vi "Time.vi"(8 "error in (no error)":errorcluster, 10 "Control In":T2={"I-O.lvclass"=refnum, "Gantry"=refnum, "Dispenser"="COM1"}, 11 "Sensor Dispense in":refnum<class "Sensor Dispense.lvclass">) -> (0 "error out":errorcluster, 1 "Timing Data":i32[](array[numeric]), 2 "Control Out":T2={"I-O.lvclass"=refnum, "Gantry"=refnum, "Dispenser"="COM1"}, 3 "Sensor Dispense out":refnum<class "Sensor Dispense.lvclass">)   [LabVIEW 2021, in "Sensor Dispense.lvclass"]
uses:
  Projects/Sensor Dispense.lvclass
  C:/Users/HEP/Documents/GitHub/Gantry/UCSB-Gantry-HEP-main/Classes/Routine/Dispense/Dispense.lvclass
  Controller/Controllers.ctl
  Controller/I-O/I-O.lvclass
  C:/Program Files (x86)/Aerotech/A3200/LabVIEW/2010/Bin/Aerotech.A3200.dll
  Program Files (x86)/Aerotech/A3200/LabVIEW/2010/Bin/Aerotech.A3200.dll
  TypeOfHexaboard.ctl
  Projects/Sensor Dispense.lvclass/Sensor Dispense.ctl
  Controller/Motion/Motion.lvclass
  Controller/Motion/A3200/A3200.lvclass
  Controller/Controller.lvclass
  Routine.lvclass
panel:
  in  "Type of Hexaboard":T1
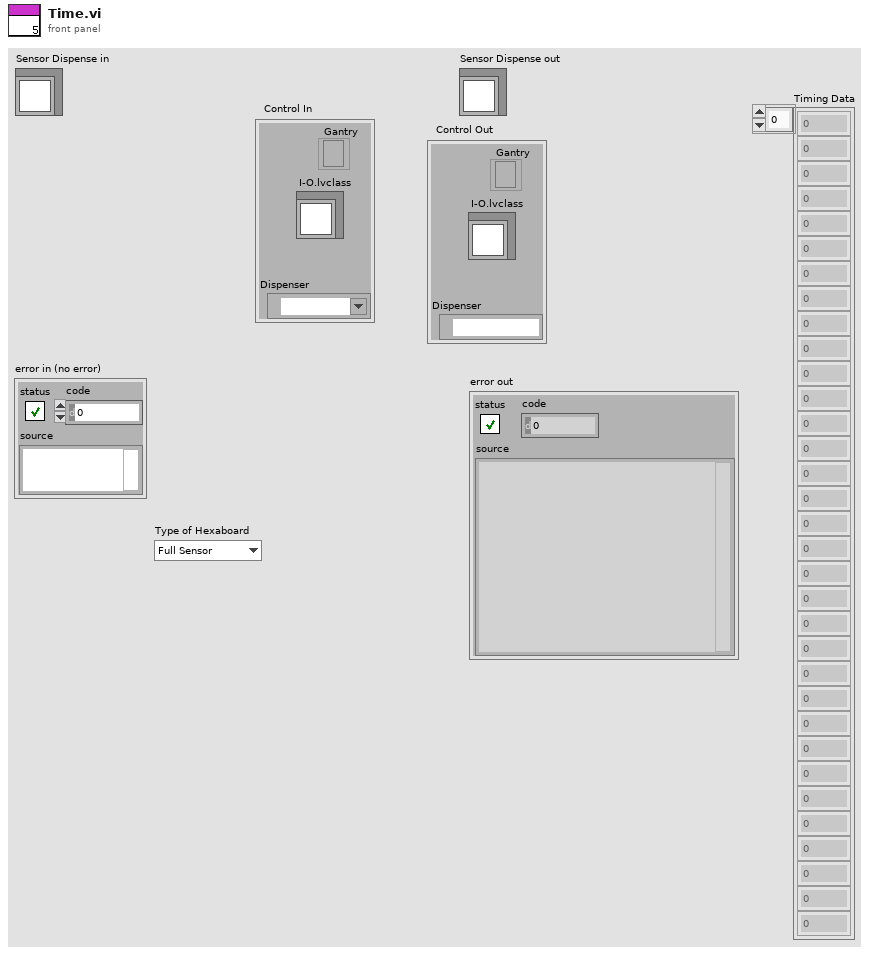
[diagram p1: front panel]
types:
  T1 = typedef "Routine.lvclass/TypeOfHexaboard.ctl" = enum16{"Full Sensor", "Full PCB", "Right Partial PCB", "Right Partial Sensor", "Al Dummy Right Partial Sensor"}
  T2 = typedef "Controller.lvclass/Controllers.ctl" = cluster{"I-O.lvclass":refnum<class "I-O.lvclass">, "Gantry":refnum<k24>, "Dispenser":refnum<visa-resource-name>}
  T3 = cluster{"Endpoints":dbl[][], "Center":dbl[], "CW/CCW":dbl, "Dispense Type":enum16{"N-gon", "Square", "Arc", "Dot", "Line", "Circle"}}[]
  T4 = cluster{"Endpoints":dbl[][], "Center":dbl[], "CW/CCW":dbl, "Dispense Type":enum16{"N-gon", "Square", "Arc", "Dot", "Line", "Circle"}}
  T5 = enum16{"N-gon", "Square", "Arc", "Dot", "Line", "Circle"}
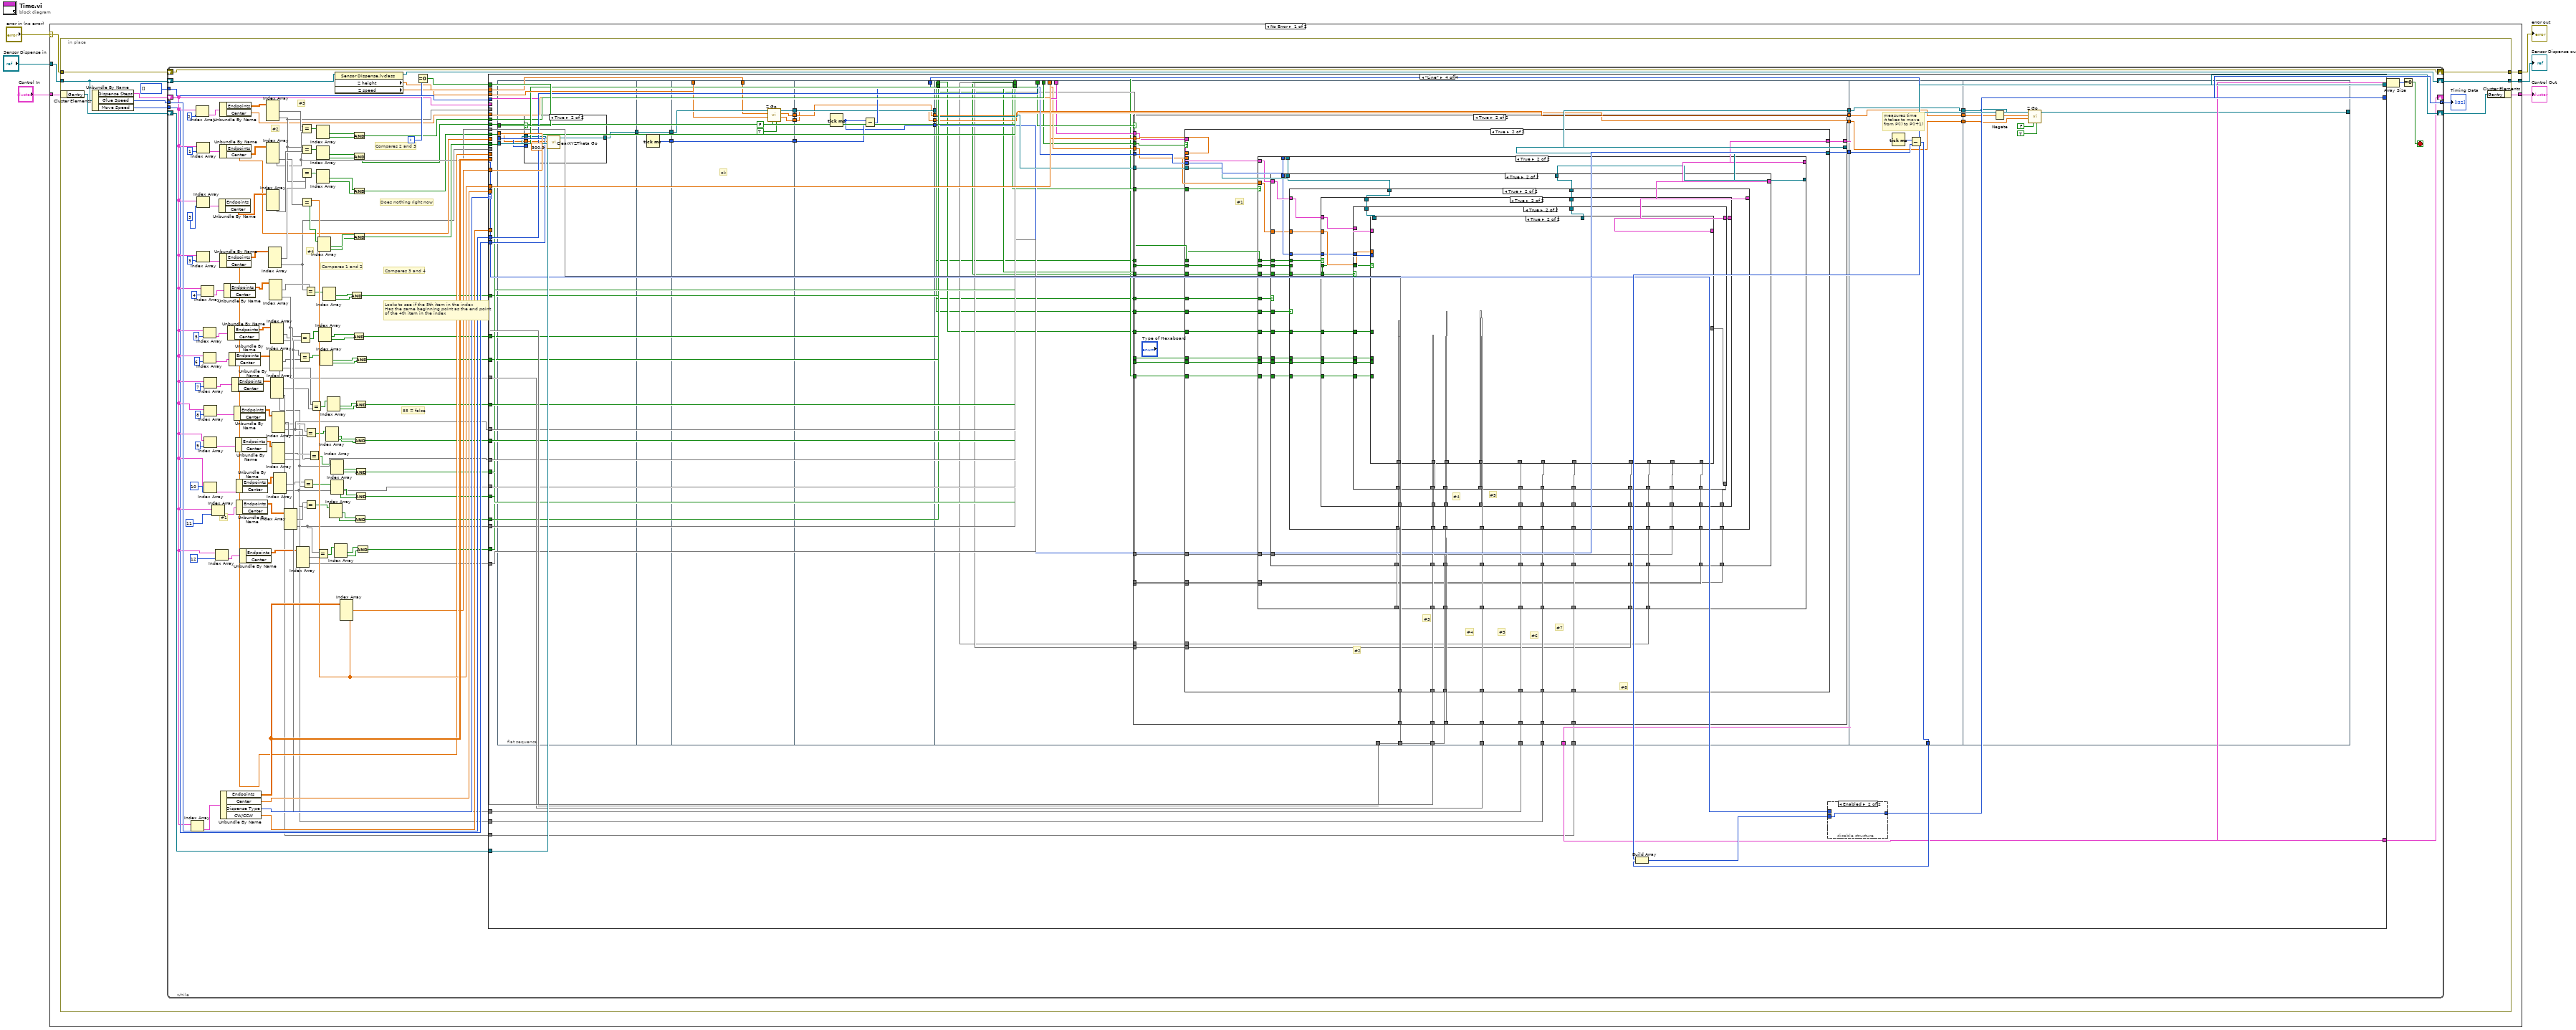
[diagram p0: block diagram]
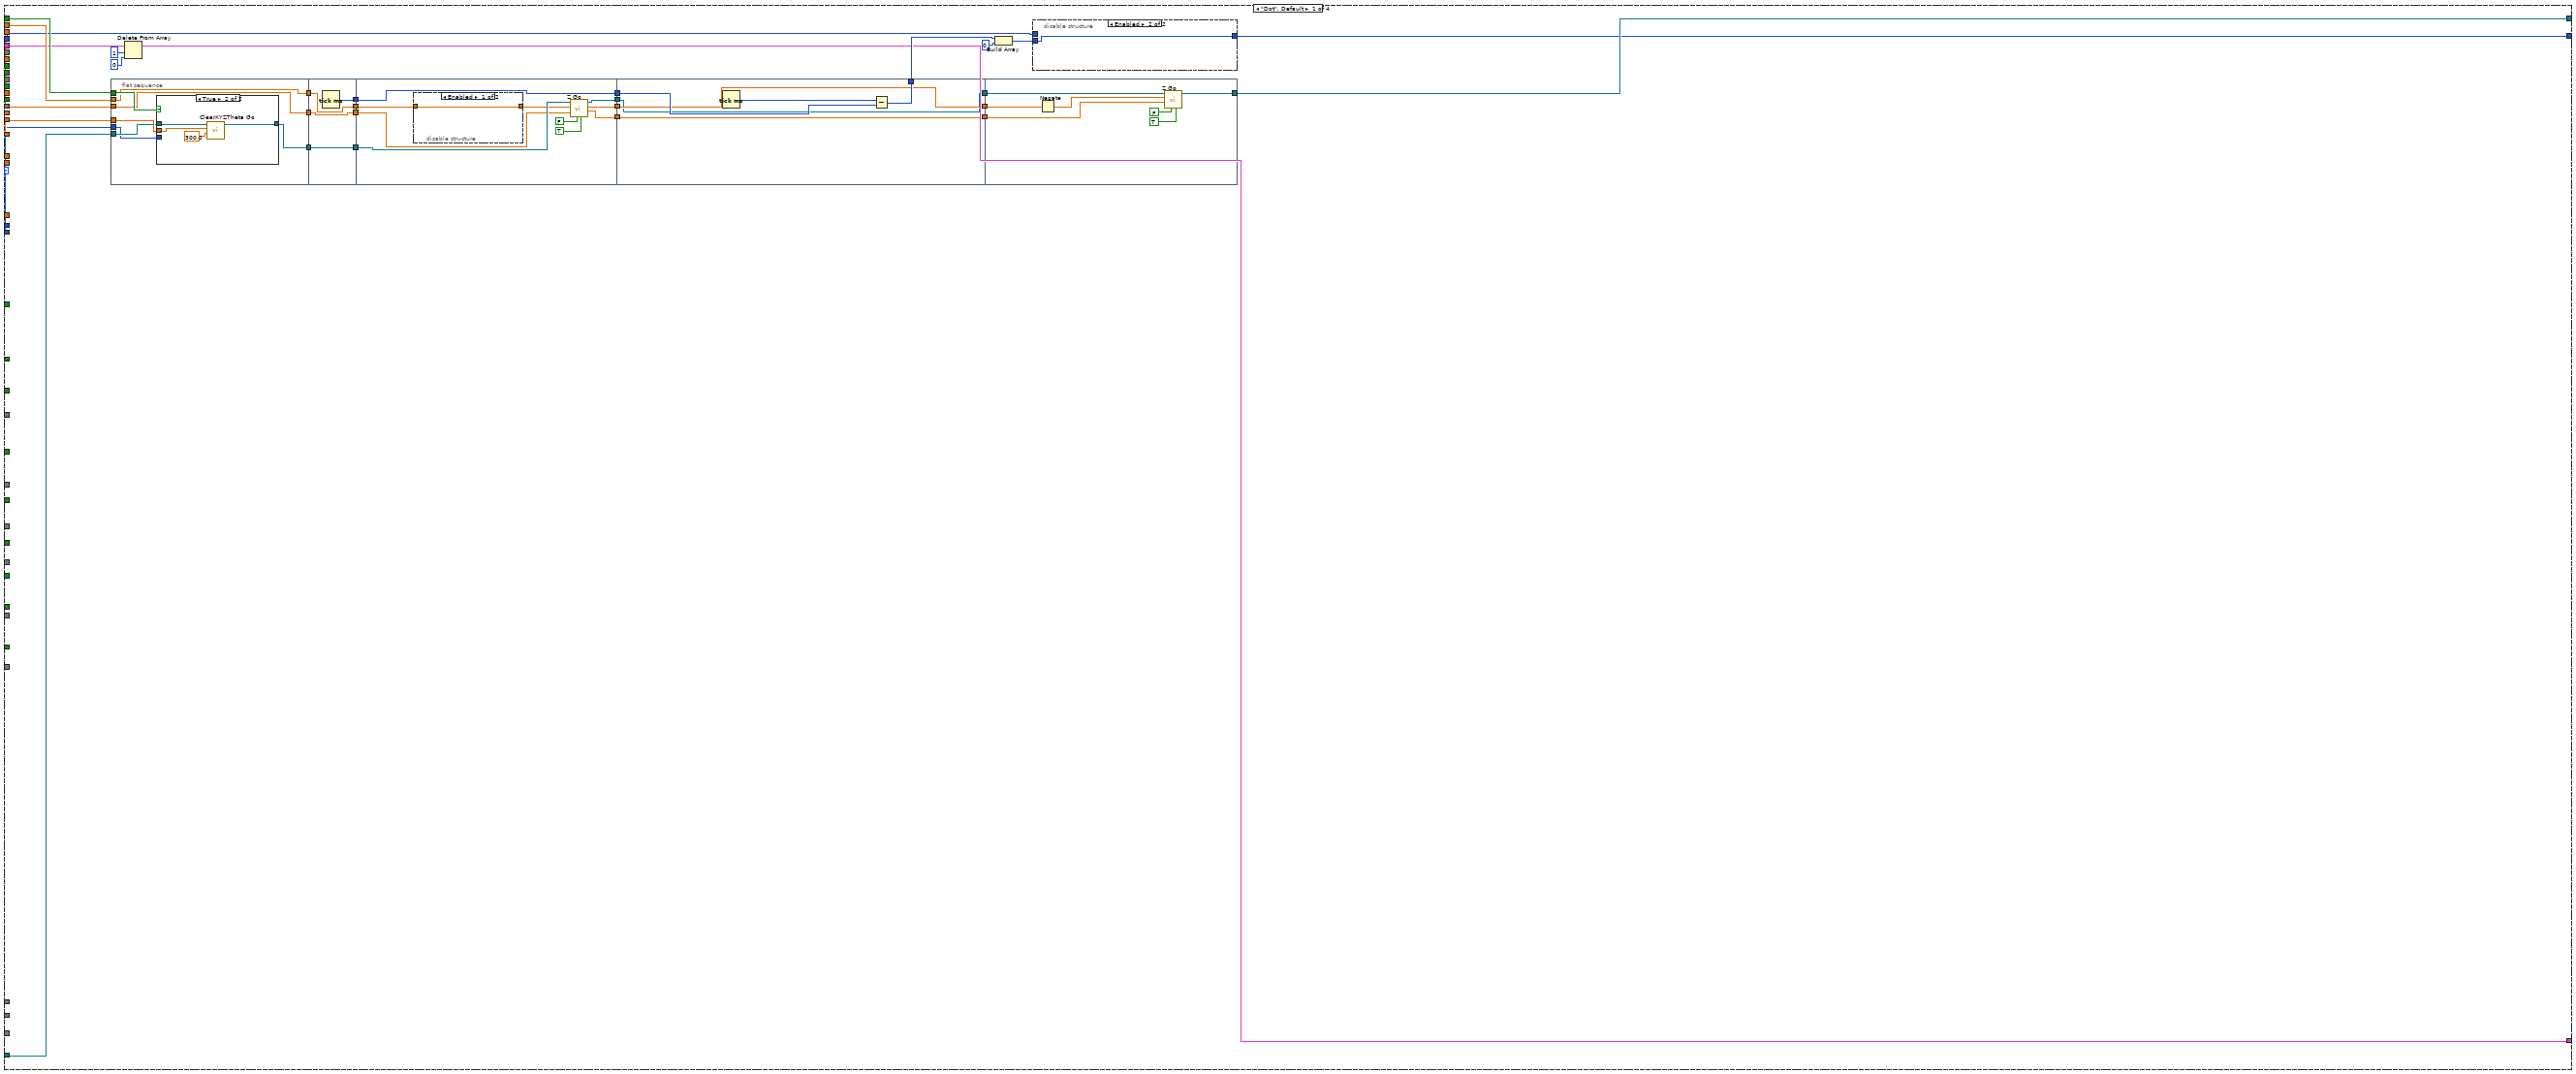
[diagram p2: hidden frame]
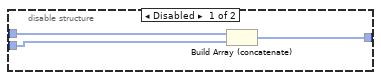
[diagram p3: hidden frame]
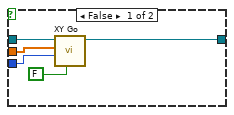
[diagram p4: hidden frame]
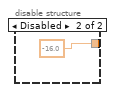
[diagram p5: hidden frame]
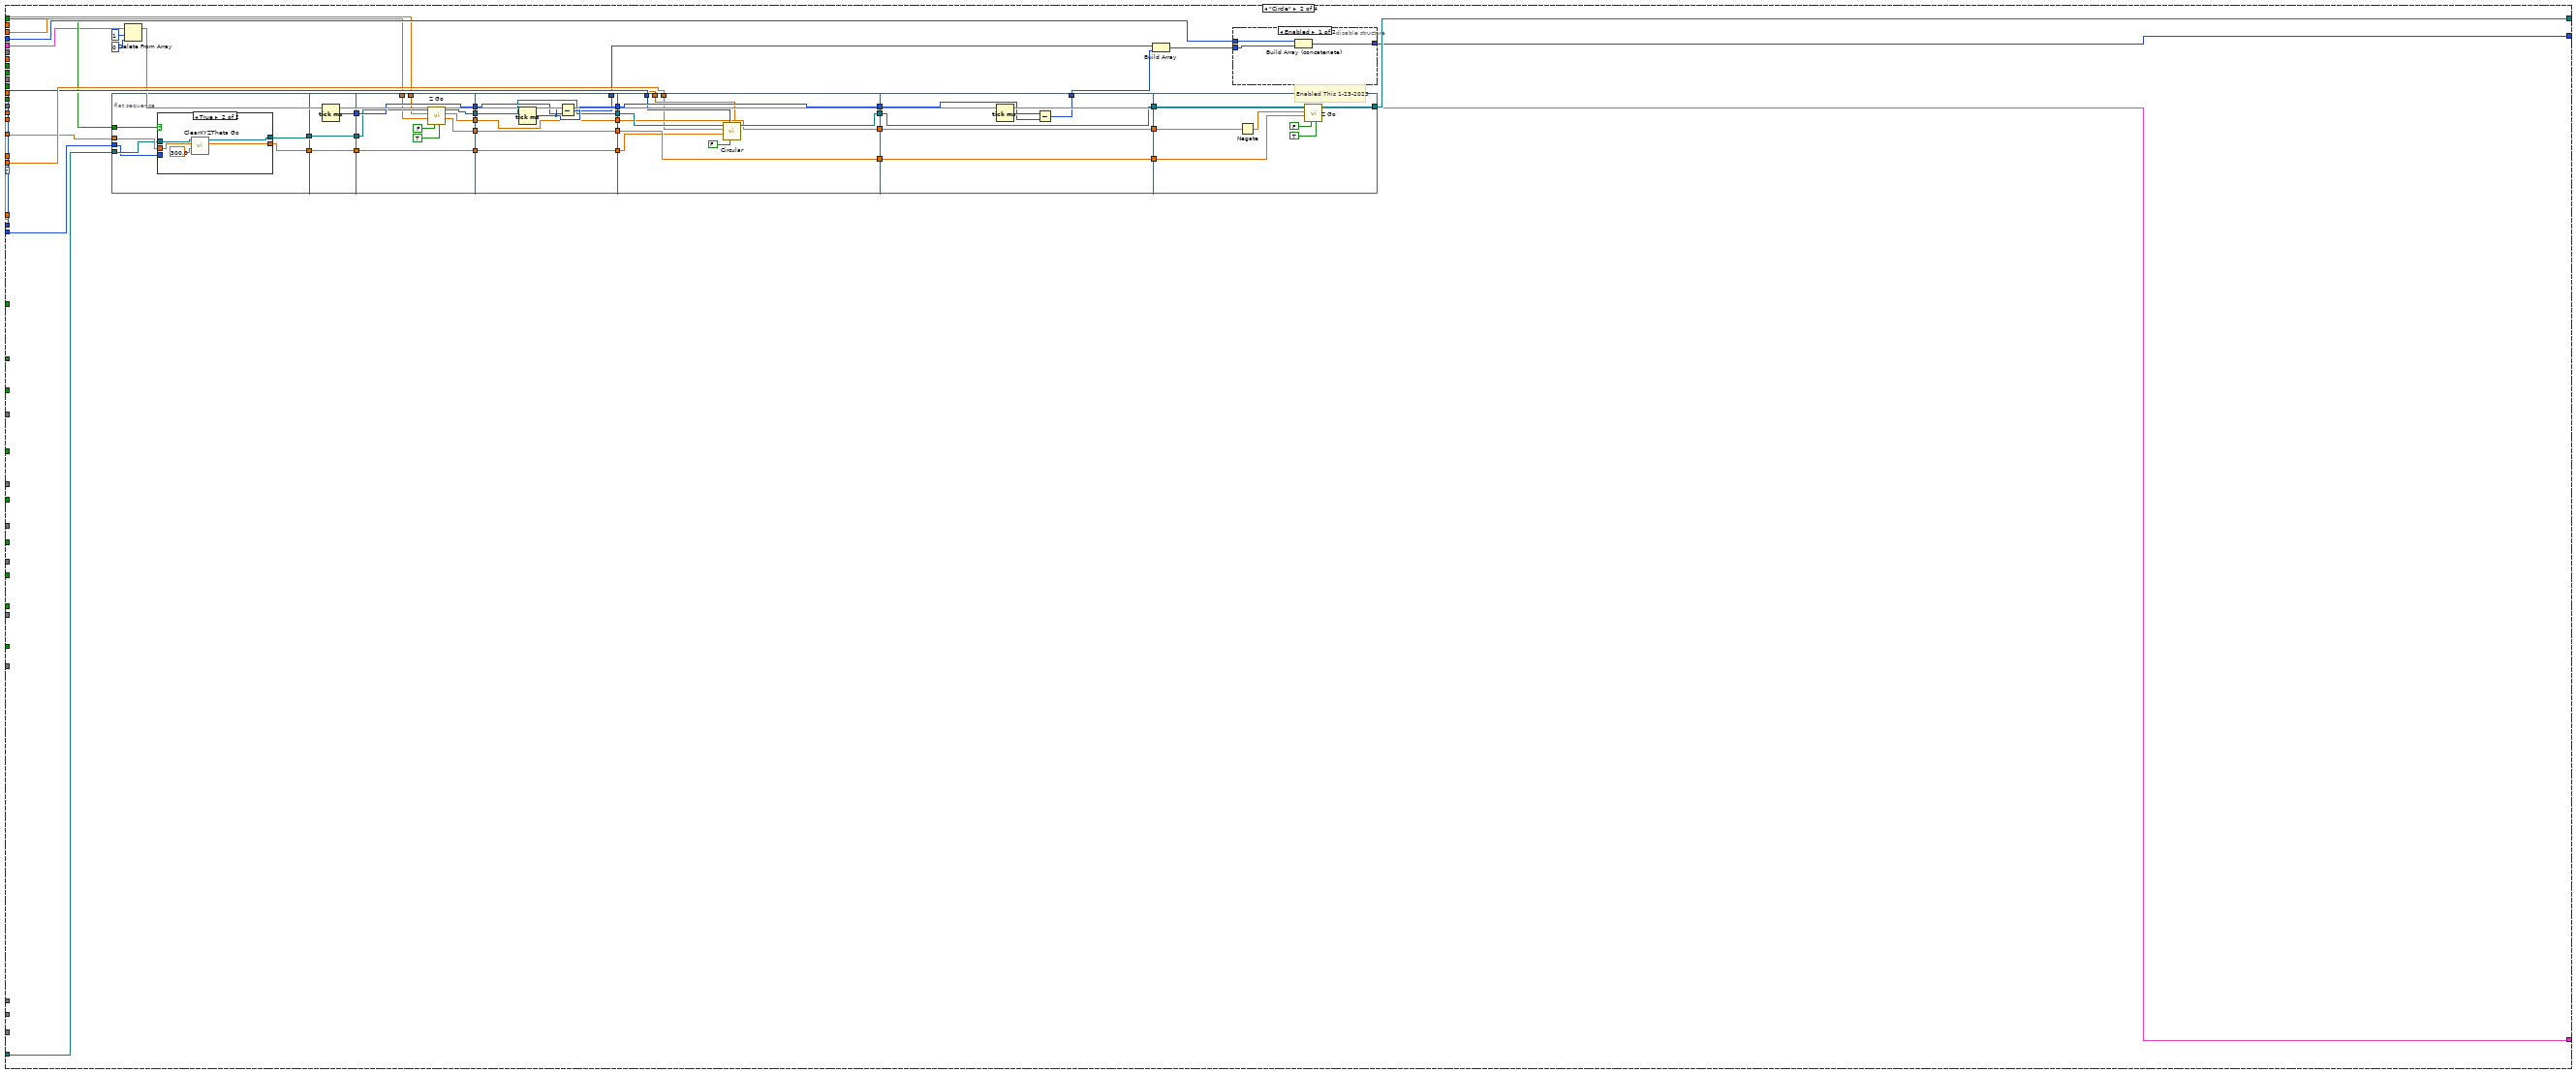
[diagram p6: hidden frame]
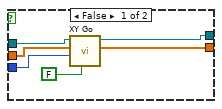
[diagram p8: hidden frame]
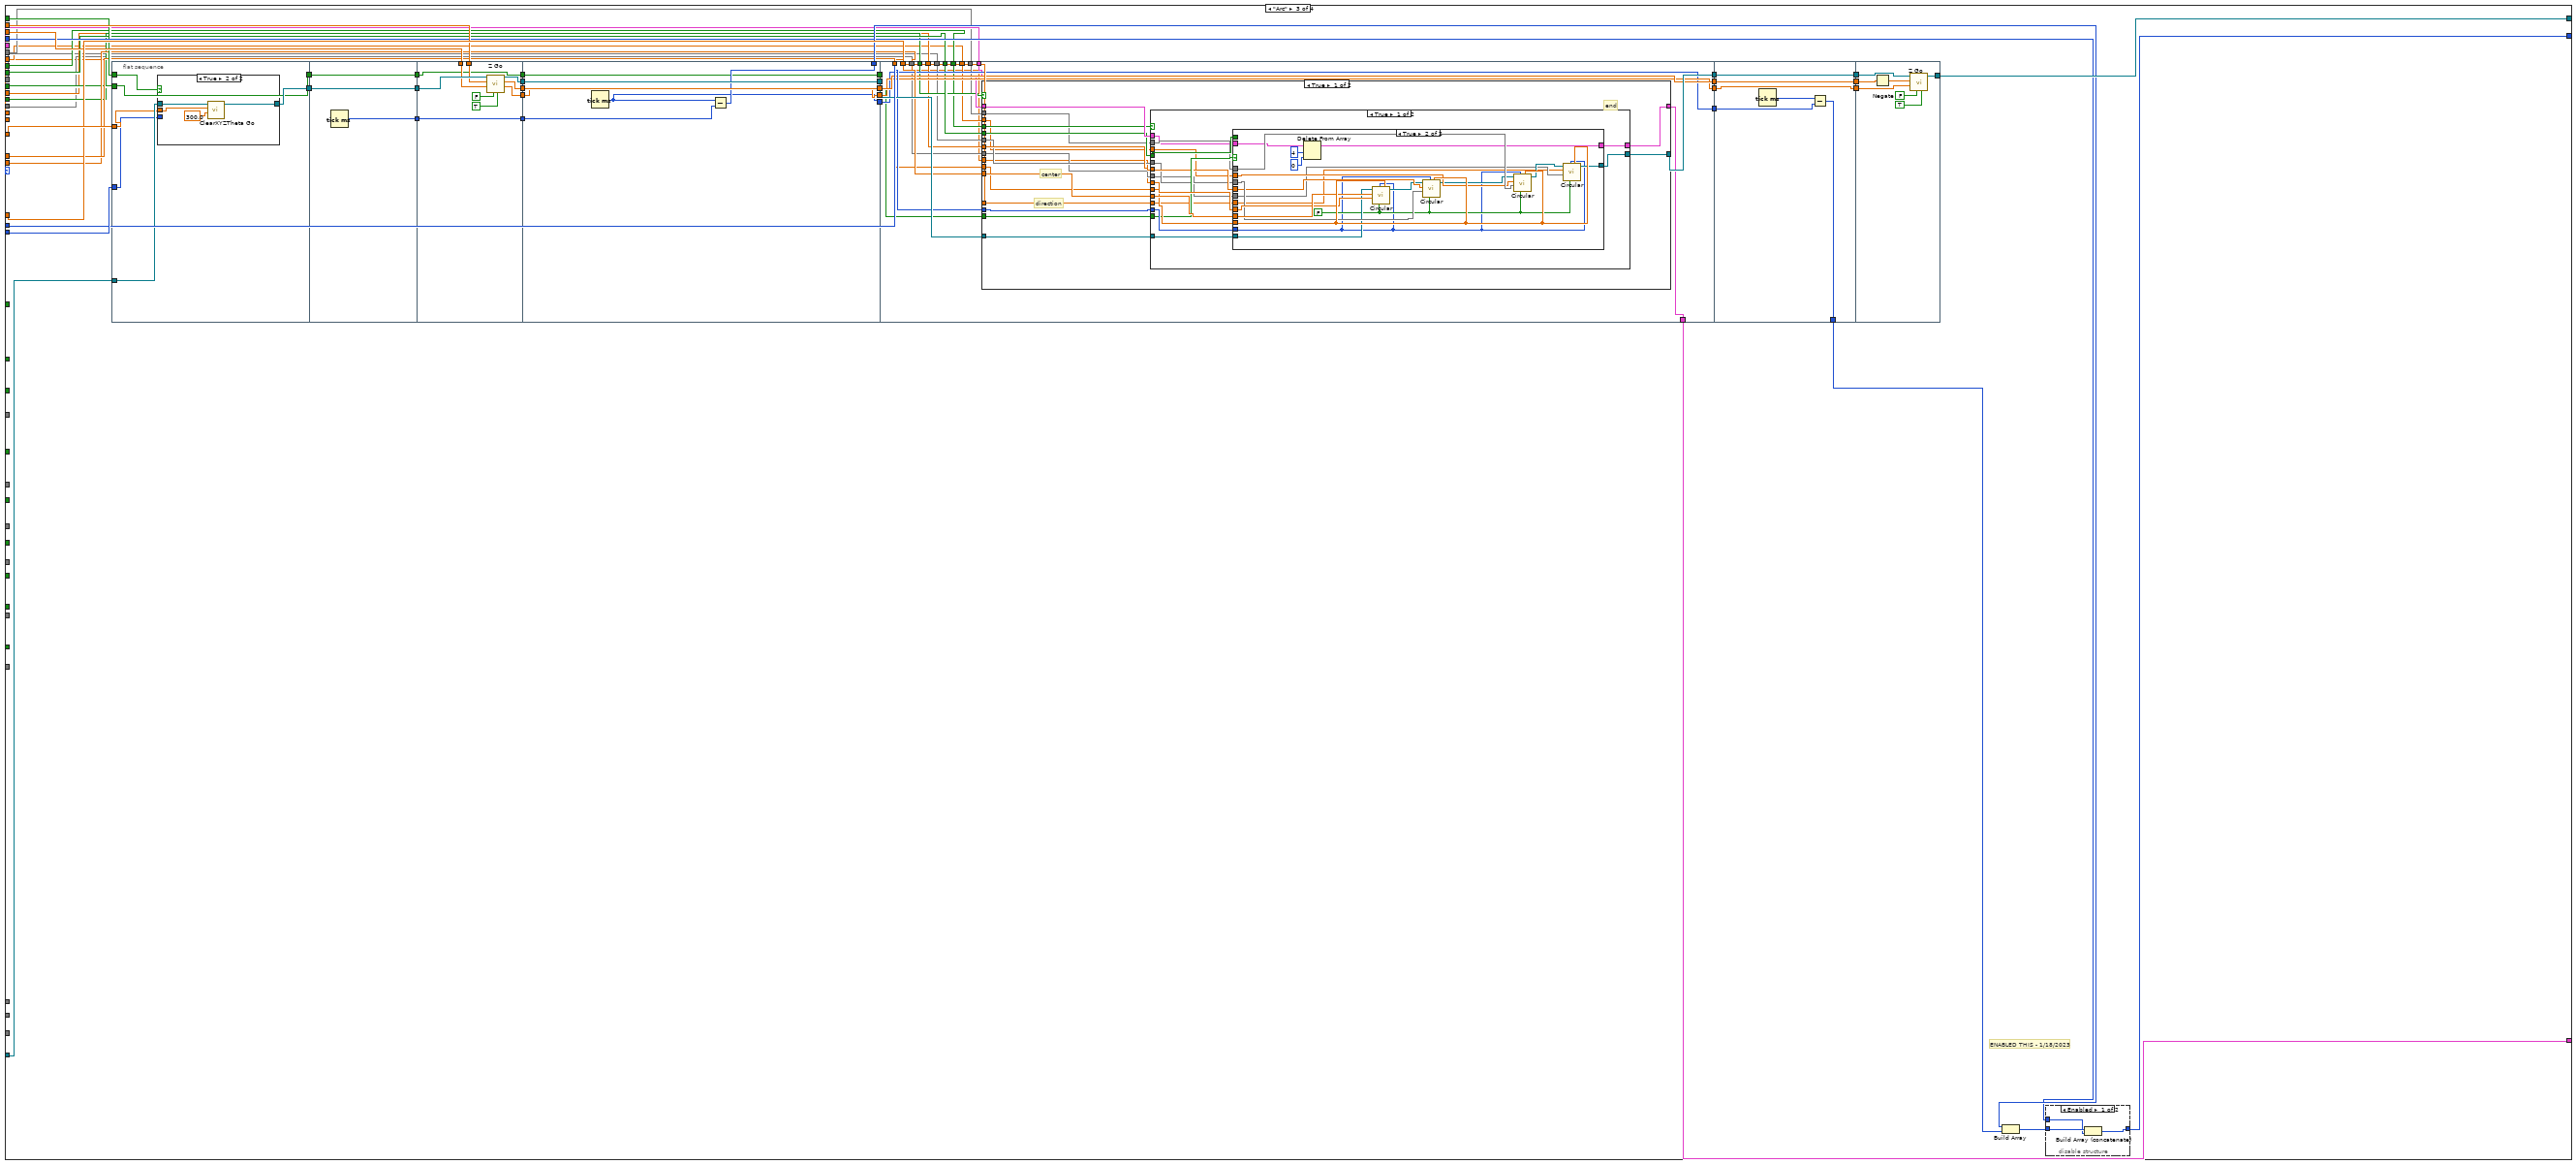
[diagram p9: hidden frame]
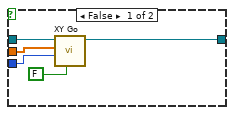
[diagram p11: hidden frame]
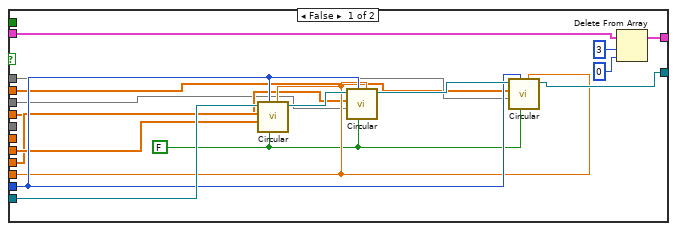
[diagram p12: hidden frame]
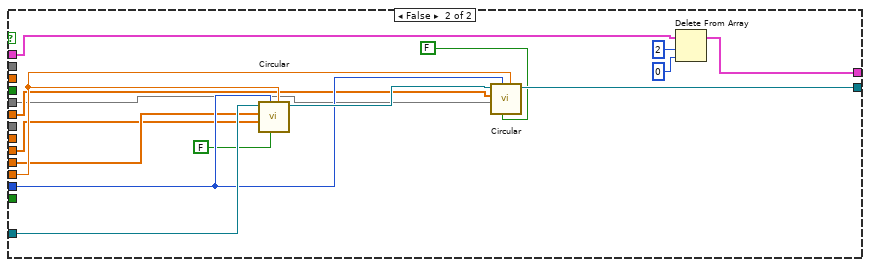
[diagram p13: hidden frame]
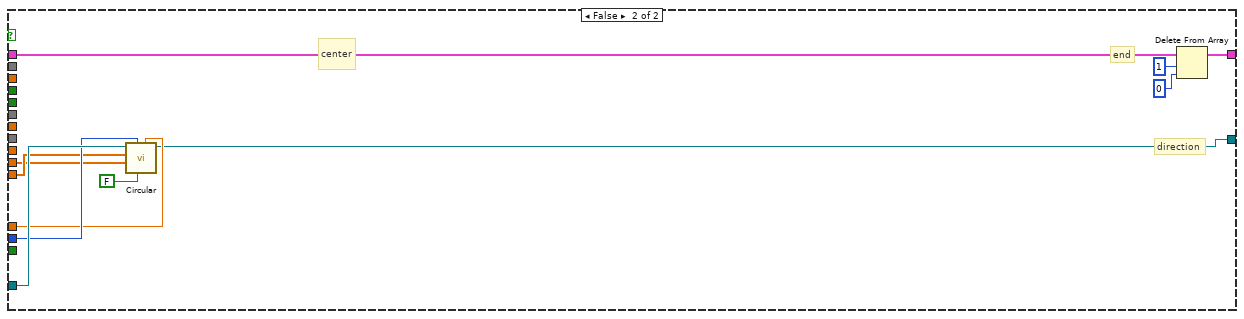
[diagram p14: hidden frame]
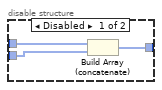
[diagram p15: hidden frame]
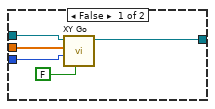
[diagram p16: hidden frame]
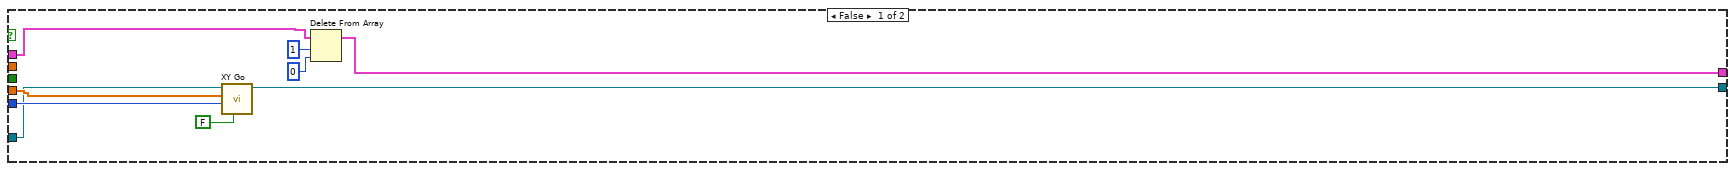
[diagram p17: hidden frame]
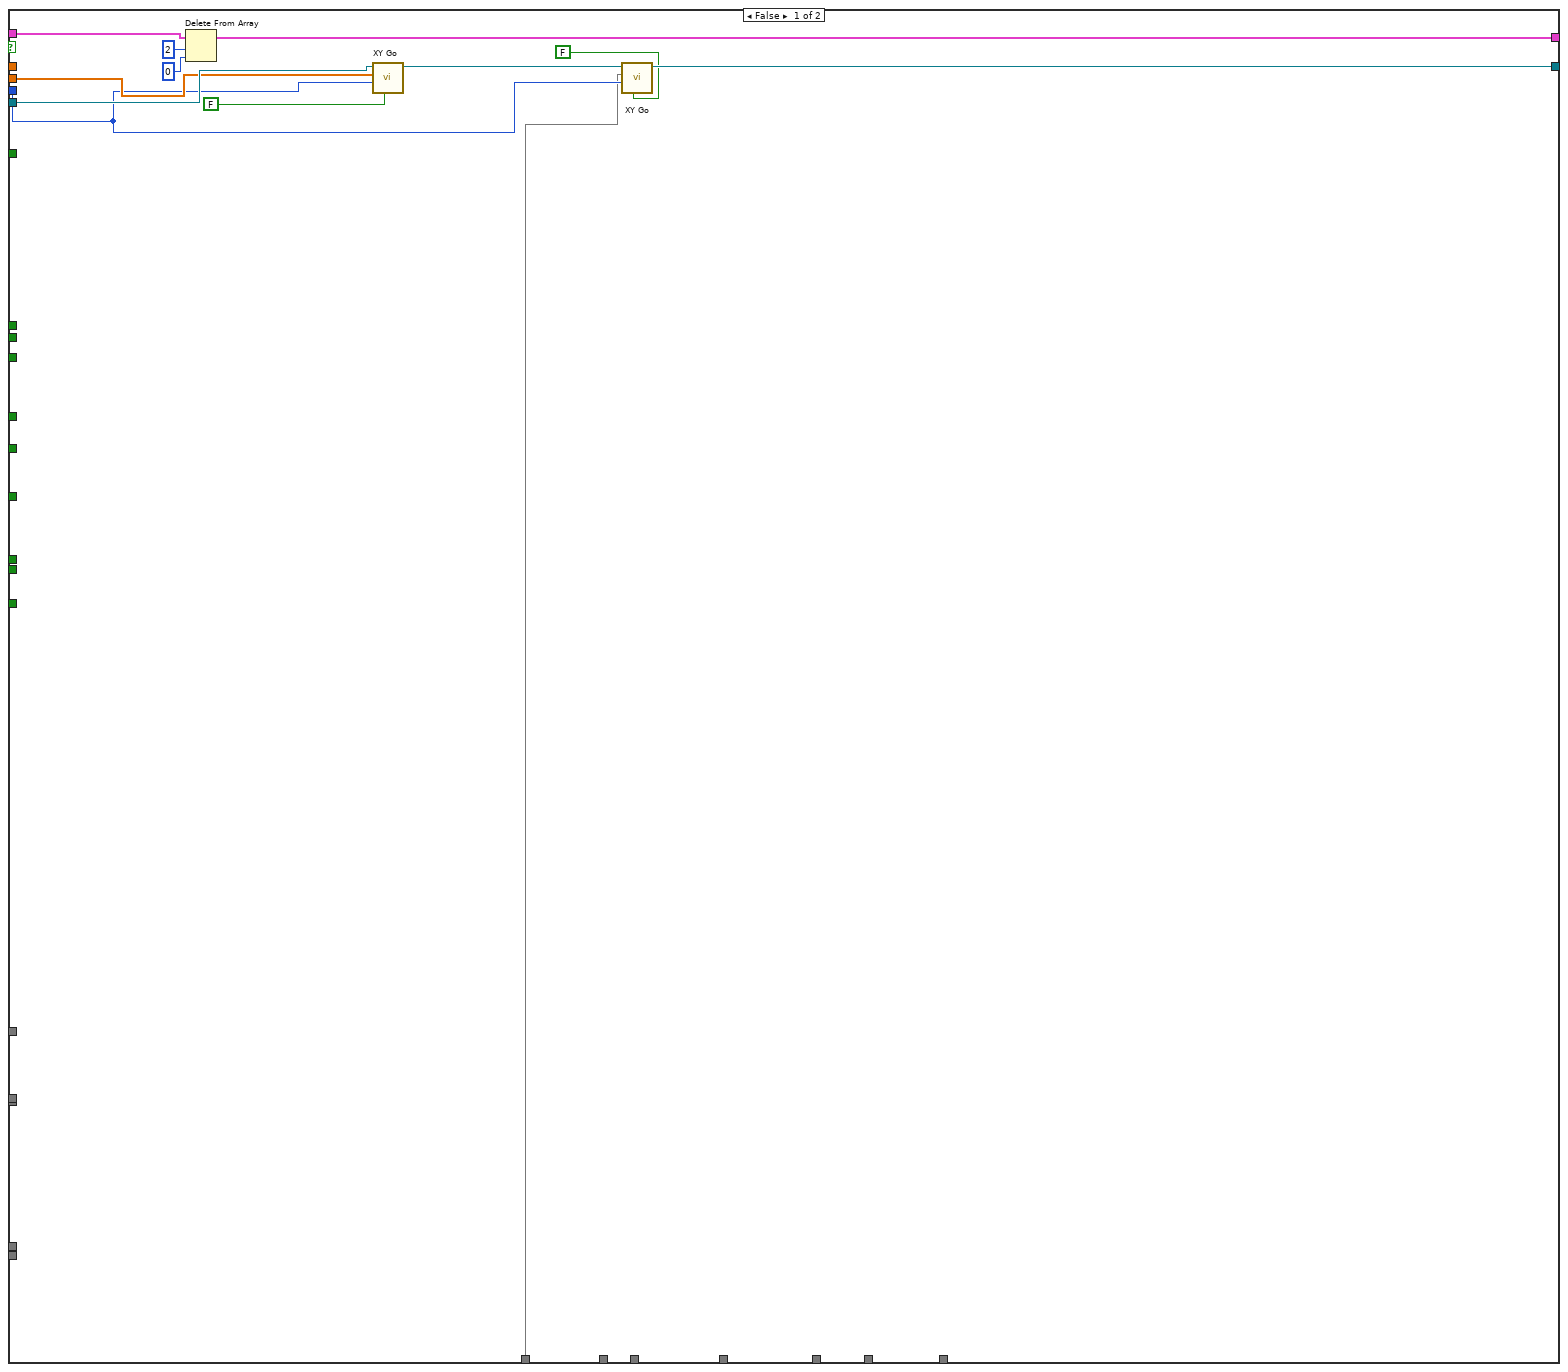
[diagram p18: hidden frame]
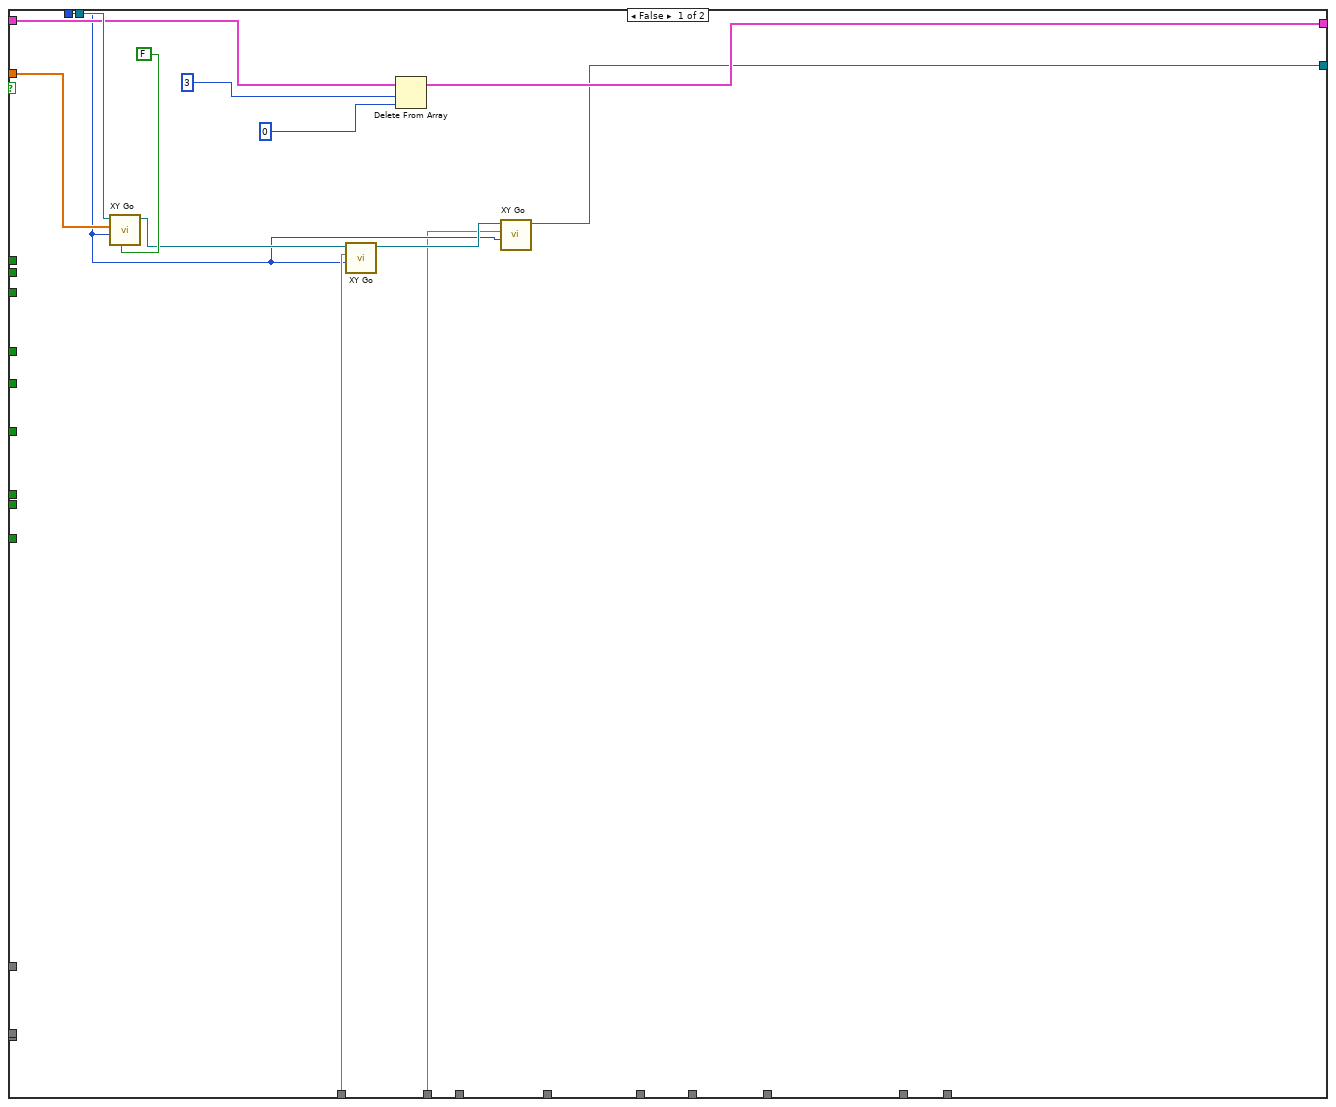
[diagram p19: hidden frame]
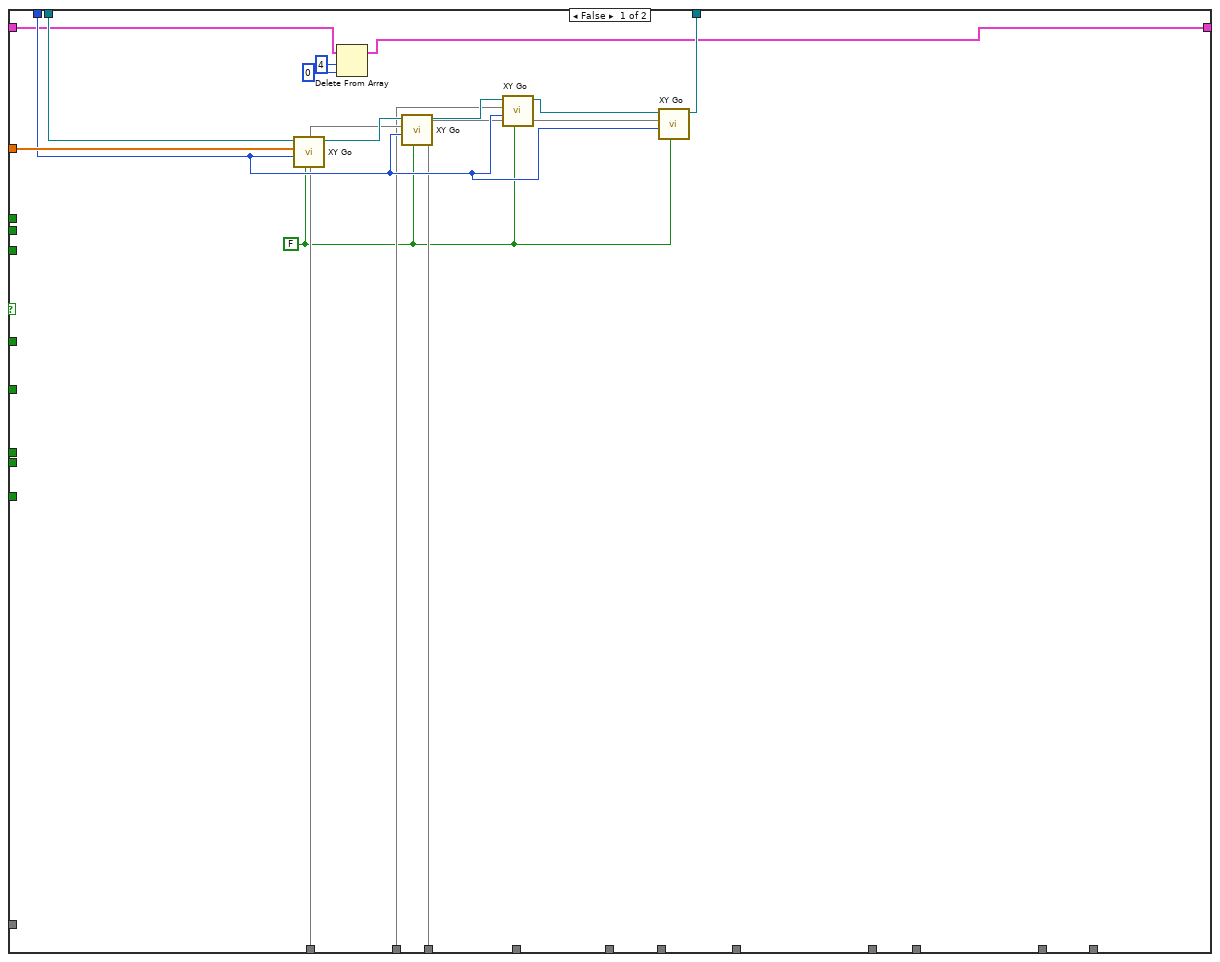
[diagram p20: hidden frame]
diagram:
  n1 = case shown="No Error" "error in (no error)" {
    selector: "error in (no error)" -> [w7 w1246]
    tunnel: "Sensor Dispense in" -> [w12 w1244]
    tunnel: [w11 w1244] -> w5
    tunnel: "Control In" -> [w10 w1245]
    tunnel: [w9 w1245] -> w3
    tunnel: [w8 w1246] -> w2
    frame No Error {
      n2 = in-place {
        in-place-border: w12 -> [w21]
        in-place-border: [w20] -> w11
        in-place-border: [w16] -> w8
        in-place-border: w7 -> [w15]
        n3 = in-place-cluster #1(w10) -> ("Gantry"=w22:refnum<k24>)
        n4 = Unbundle By Name "Unbundle By Name"(w21) -> ("Dispense Steps"=w17:T3, "Glue Speed"=w13:i32, "Move Speed"=w14:i32)
        n5 = while {
          tunnel: w14 -> [w166]
          shift-right: [w155] -> w19
          shift-left: w22 -> [w164]
          tunnel: w13 -> [w152]
          shift-right: [w162] -> w20
          shift-left: w21 -> [w163]
          shift-right: [w113] -> w16
          shift-left: w15 -> [w113]
          tunnel: i32[] [] -> [w165]
          tunnel: [w157] -> w18 mode=concatenating
          shift-right: [w115] -> _
          shift-left: w17 -> [w40]
          i -> [w161]
          stop <- w112 stop-if-true
          # "85 = false"
          # "Looks to see if the 5th item in the index\nHas the same beginning point as the end point\nof the 4th item in the index"
          # "Does nothing right now"
          # "Compares 2 and 3"
          # "Compares 3 and 4"
          # "Compares 1 and 2"
          # "#3"
          # "#2"
          # "#1"
          # "#4"
          n6 = Index Array(array=w40) -> (element=w148:T4)  [unwired: 1 in]
          n7 = Index Array "Index Array"(array=w40, index=2) -> (element=w146:T4)
          n8 = Index Array(array=w40, index=1) -> (element=w145:T4)
          n9 = Index Array(array=w40, index=3) -> (element=w147:T4)
          n10 = Index Array(array=w40, index=3) -> (element=w150:T4)
          n11 = Index Array "Index Array"(array=w40, index=4) -> (element=w105:T4)
          n12 = Index Array "Index Array"(array=w40, index=5) -> (element=w93:T4)
          n13 = Index Array "Index Array"(array=w40, index=6) -> (element=w94:T4)
          n14 = Index Array "Index Array"(array=w40, index=7) -> (element=w95:T4)
          n15 = Index Array "Index Array"(array=w40, index=8) -> (element=w70:T4)
          n16 = Index Array "Index Array"(array=w40, index=9) -> (element=w69:T4)
          n17 = Index Array "Index Array"(array=w40, index=10) -> (element=w68:T4)
          n18 = Index Array "Index Array"(array=w40, index=11) -> (element=w67:T4)
          n19 = Index Array "Index Array"(array=w40, index=12) -> (element=w66:T4)
          n20 = Unbundle By Name(w147) -> ("Endpoints"=w139:dbl[][])  [unwired: 1 out]
          n21 = Unbundle By Name(w146) -> ("Endpoints"=w140:dbl[][], "Center"=w117:dbl[])
          n22 = Unbundle By Name(w145) -> ("Endpoints"=w138:dbl[][], "Center"=w109:dbl[])
          n23 = Unbundle By Name(w150) -> ("Endpoints"=w141:dbl[][], "Center"=w116:dbl[])
          n24 = Unbundle By Name(w148) -> ("Endpoints"=w154:dbl[][], "Center"=w153:dbl[], "Dispense Type"=w156:T5, "CW/CCW"=w151:dbl)
          n25 = Unbundle By Name(w105) -> ("Endpoints"=w101:dbl[][])  [unwired: 1 out]
          n26 = Unbundle By Name(w93) -> ("Endpoints"=w92:dbl[][])  [unwired: 1 out]
          n27 = Unbundle By Name(w94) -> ("Endpoints"=w91:dbl[][])  [unwired: 1 out]
          n28 = Unbundle By Name(w95) -> ("Endpoints"=w90:dbl[][])  [unwired: 1 out]
          n29 = Unbundle By Name(w70) -> ("Endpoints"=w65:dbl[][])  [unwired: 1 out]
          n30 = Unbundle By Name(w69) -> ("Endpoints"=w60:dbl[][])  [unwired: 1 out]
          n31 = Unbundle By Name(w68) -> ("Endpoints"=w54:dbl[][])  [unwired: 1 out]
          n32 = Unbundle By Name(w67) -> ("Endpoints"=w48:dbl[][])  [unwired: 1 out]
          n33 = Unbundle By Name(w66) -> ("Endpoints"=w42:dbl[][])  [unwired: 1 out]
          n34 = Index Array(array=w140) -> (element #1=w130:dbl[], element #2=w118:dbl[])  [unwired: 4 in]
          n35 = Index Array(array=w138) -> (element #1=w121:dbl[], element #2=w111:dbl[])  [unwired: 4 in]
          n36 = Index Array(array=w139) -> (element #1=w134:dbl[])  [unwired: 4 in, 1 out]
          n37 = Index Array(array=w141) -> (element #1=w123:dbl[], element #2=w99:dbl[])  [unwired: 4 in]
          n38 = Index Array(array=w101) -> (element #1=w100:dbl[], element #2=w89:dbl[])  [unwired: 4 in]
          n39 = Index Array(array=w91) -> (element #1=w83:dbl[], element #2=w38:dbl[])  [unwired: 4 in]
          n40 = Index Array(array=w92) -> (element #1=w88:dbl[], element #2=w84:dbl[])  [unwired: 4 in]
          n41 = Index Array(array=w90) -> (element #1=w79:dbl[], element #2=w39:dbl[])  [unwired: 4 in]
          n42 = Index Array(array=w65) -> (element #1=w64:dbl[], element #2=w58:dbl[])  [unwired: 4 in]
          n43 = Index Array(array=w60) -> (element #1=w59:dbl[], element #2=w53:dbl[])  [unwired: 4 in]
          n44 = Index Array(array=w54) -> (element #1=w52:dbl[], element #2=w46:dbl[])  [unwired: 4 in]
          n45 = Index Array(array=w48) -> (element #1=w47:dbl[], element #2=w32:dbl[])  [unwired: 4 in]
          n46 = Index Array(array=w42) -> (element #1=w33:dbl[], element #2=w41:dbl[])  [unwired: 4 in]
          n47 = Equal?(x=w84, y=w83) -> (x = y?=w82:bool[])
          n48 = Equal?(x=w89, y=w88) -> (x = y?=w87:bool[])
          n49 = Equal?(x=w111, y=w130) -> (x = y?=w129:bool[])
          n50 = Equal?(x=w118, y=w134) -> (x = y?=w133:bool[])
          n51 = Equal?(x=w118, y=w123) -> (x = y?=w137:bool[])
          n52 = Equal?(x=w52, y=w53) -> (x = y?=w51:bool[])
          n53 = Equal?(x=w99, y=w100) -> (x = y?=w102:bool[])
          n54 = Equal?(x=w39, y=w64) -> (x = y?=w63:bool[])
          n55 = Equal?(x=w47, y=w46) -> (x = y?=w45:bool[])
          n56 = Equal?(x=w59, y=w58) -> (x = y?=w57:bool[])
          n57 = Equal?(x=w38, y=w79) -> (x = y?=w78:bool[])
          n58 = Index Array(array=w129) -> (element #1=w128:bool, element #2=w127:bool)  [unwired: 2 in]
          n59 = Index Array(array=w133) -> (element #1=w132:bool, element #2=w131:bool)  [unwired: 2 in]
          n60 = Index Array(array=w137) -> (element #1=w136:bool, element #2=w135:bool)  [unwired: 2 in]
          n61 = Equal?(x=w32, y=w33) -> (x = y?=w31:bool[])
          n62 = Index Array(array=w87) -> (element #1=w86:bool, element #2=w85:bool)  [unwired: 2 in]
          n63 = Index Array(array=w82) -> (element #1=w81:bool, element #2=w80:bool)  [unwired: 2 in]
          n64 = Index Array(array=w102) -> (element #1=w104:bool, element #2=w103:bool)  [unwired: 2 in]
          n65 = Index Array(array=w63) -> (element #1=w62:bool, element #2=w61:bool)  [unwired: 2 in]
          n66 = Index Array(array=w78) -> (element #1=w77:bool, element #2=w76:bool)  [unwired: 2 in]
          n67 = Index Array(array=w45) -> (element #1=w44:bool, element #2=w43:bool)  [unwired: 2 in]
          n68 = Index Array(array=w57) -> (element #1=w56:bool, element #2=w55:bool)  [unwired: 2 in]
          n69 = Index Array(array=w51) -> (element #1=w50:bool, element #2=w49:bool)  [unwired: 2 in]
          n70 = Index Array(array=w31) -> (element #1=w30:bool, element #2=w29:bool)  [unwired: 2 in]
          n71 = property class="Sensor Dispense.lvclass"(reference=w163) -> (reference out=w162:refnum<class "Sensor Dispense.lvclass">, "Z height"=w159:dbl, "Z speed"=w158:dbl)  [unwired: 1 in, 1 out]
          n72 = Index Array(array=w154) -> (element #1=w110:dbl[], element #2=w122:dbl[])  [unwired: 4 in]
          n73 = Equal?(x=w122, y=w121) -> (x = y?=w126:bool[])
          n74 = Index Array(array=w126) -> (element #1=w125:bool, element #2=w124:bool)  [unwired: 2 in]
          n75 = And(x=w104, y=w103) -> (x .and. y?=w25:bool)
          n76 = And(x=w86, y=w85) -> (x .and. y?=w24:bool)
          n77 = And(x=w128, y=w127) -> (x .and. y?=w120:bool)
          n78 = And(x=w132, y=w131) -> (x .and. y?=w107:bool)
          n79 = And(x=w136, y=w135) -> (x .and. y?=w108:bool)
          n80 = And(x=w125, y=w124) -> (x .and. y?=w119:bool)
          n81 = And(x=w62, y=w61) -> (x .and. y?=w36:bool)
          n82 = And(x=w44, y=w43) -> (x .and. y?=w28:bool)
          n83 = And(x=w77, y=w76) -> (x .and. y?=w37:bool)
          n84 = And(x=w56, y=w55) -> (x .and. y?=w35:bool)
          n85 = And(x=w50, y=w49) -> (x .and. y?=w34:bool)
          n86 = And(x=w81, y=w80) -> (x .and. y?=w26:bool)
          n87 = And(x=w30, y=w29) -> (x .and. y?=w27:bool)
          n88 = Equal To 0?(x=w161) -> (x = 0?=w160:bool)
          n89 = case shown="\"Line\"" w156 {
            tunnel: w153 -> [_ w274 w375 _]
            tunnel: w164 -> [w192 w275 w400 w629]
            tunnel: w166 -> [w176 w263 w398 w627]
            tunnel: [w177 w282 w387 w603] -> w155
            tunnel: w152 -> [_ w273 w397 w617]
            tunnel: w151 -> [_ w272 w396 _]
            tunnel: w165 -> [w173 w269 w379 w601]
            tunnel: [w171 w267 w378 w599] -> w157
            tunnel: w110 -> [w193 w262 w399 w628]
            tunnel: w158 -> [w186 w265 w394 w622]
            tunnel: w159 -> [w189 w266 w395 w623]
            tunnel: w160 -> [w194 w264 w377 w626]
            tunnel: w154 -> [_ _ _ _]
            tunnel: w122 -> [_ _ w376 w598]
            tunnel: w40 -> [w170 w249 w366 w594]
            tunnel: [w169 w248 w365 w593] -> w115
            tunnel: w108 -> [_ _ w360 w590]
            tunnel: w107 -> [_ _ w359 w589]
            tunnel: w120 -> [_ _ w358 w596]
            tunnel: w119 -> [_ _ w357 w597]
            tunnel: w109 -> [_ _ w356 _]
            tunnel: w111 -> [_ _ w355 w592]
            tunnel: w118 -> [_ _ w354 w591]
            tunnel: w117 -> [_ _ w353 w595]
            tunnel: w99 -> [_ _ w352 w588]
            tunnel: w116 -> [_ _ w351 _]
            tunnel: w89 -> [_ _ _ w587]
            tunnel: w84 -> [_ _ _ w586]
            tunnel: w38 -> [_ _ _ w585]
            tunnel: w39 -> [_ _ _ w584]
            tunnel: w58 -> [_ _ _ w583]
            tunnel: w53 -> [_ _ _ w582]
            tunnel: w46 -> [_ _ _ w581]
            tunnel: w32 -> [_ _ _ w580]
            tunnel: w41 -> [_ _ _ w579]
            tunnel: w37 -> [_ _ _ w578]
            tunnel: w36 -> [_ _ _ w577]
            tunnel: w35 -> [_ _ _ w576]
            tunnel: w34 -> [_ _ _ w575]
            tunnel: w28 -> [_ _ _ w574]
            tunnel: w27 -> [_ _ _ w573]
            tunnel: w26 -> [_ _ _ w572]
            tunnel: w25 -> [_ _ _ w571]
            tunnel: w24 -> [_ _ _ w570]
            frame "Dot", Default {
              n90 = flat-sequence {
                tunnel: w194 -> [w207]
                tunnel: w193 -> [w206]
                tunnel: w192 -> [w205]
                tunnel: [w204] -> w190
                tunnel: w189 -> [w203]
                tunnel: [w203] -> w187
                tunnel: w186 -> [w202]
                tunnel: [w202] -> w184
                tunnel: w176 -> [w201]
                tunnel: [w220] -> w196
                tunnel: [w219] -> w191
                tunnel: w190 -> [w219]
                tunnel: [w218] -> w188
                tunnel: w187 -> [w218]
                tunnel: [w217] -> w185
                tunnel: w184 -> [w217]
                tunnel: [w230] -> w195
                tunnel: w196 -> [w230]
                tunnel: w191 -> [w229]
                tunnel: w188 -> [w222]
                tunnel: w185 -> [w228]
                tunnel: [w227] -> w182
                tunnel: [w226] -> w180
                tunnel: [w225] -> w178
                tunnel: w195 -> [w238]
                tunnel: [w236] -> w175
                tunnel: [w235] -> w183
                tunnel: w182 -> [w235]
                tunnel: [w234] -> w181
                tunnel: w180 -> [w234]
                tunnel: [w233] -> w179
                tunnel: w178 -> [w233]
                tunnel: w183 -> [w245]
                tunnel: w181 -> [w243]
                tunnel: w179 -> [w242]
                tunnel: [w241] -> w177
                frame #0 {
                  n91 = case shown="True" w207 {
                    tunnel: w206 -> [w210 w216]
                    tunnel: w205 -> [w212 w215]
                    tunnel: [w211 w214] -> w204
                    tunnel: w201 -> [w209 _]
                    frame False {
                      n92 = call "XY Go.vi"("return immediately"=FALSE, "Speed"=w209, "XY In"=w210, "Gantry In"=w212) -> ("Gantry Out"=w211:refnum<k24>)  [unwired: 5 in, 2 out]
                    }
                    frame True {
                      n93 = call "ClearXYZTheta Go.vi"("Speed"=300.0, "XYZTheta In"=w216, "Gantry In"=w215) -> ("Gantry Out"=w214:refnum<k24>)  [unwired: 6 in, 2 out]
                    }
                  }
                }
                frame #1 {
                  n94 = Tick Count (ms)() -> (millisecond timer value=w220:u32)
                }
                frame #2 {
                  n95 = disable-structure shown="Enabled" {
                    disable-tunnel: w222 -> [w231 _]
                    disable-tunnel: [w231 -16.0 ("Z height")] -> w221
                    frame Enabled {
                    }
                    frame Disabled {
                    }
                  }
                  n96 = call "Z Go.vi"("Increment"=TRUE, "Return Immediately"=FALSE, "Speed In"=w228, "Position In"=w221, "Gantry In"=w229) -> ("Speed Out"=w226:dbl, "Position Out"=w227:dbl, "Gantry Out"=w225:refnum<k24>)  [unwired: 3 in, 1 out]
                }
                frame #3 {
                  n97 = Tick Count (ms)() -> (millisecond timer value=w237:u32)
                  n98 = Subtract(x=w237, y=w238) -> (x-y=w236:u32)
                }
                frame #4 {
                  n99 = Negate(x=w245) -> (-x=w244:dbl)
                  n100 = call "Z Go.vi"("Increment"=TRUE, "Return Immediately"=FALSE, "Speed In"=w243, "Position In"=w244, "Gantry In"=w242) -> ("Gantry Out"=w241:refnum<k24>)  [unwired: 3 in, 3 out]
                }
              }
              n101 = Delete From Array(array=w170, length=1, index=0) -> (array with subset deleted=w169:T3)  [unwired: 1 out]
              n102 = Build Array(w175, u32 0 ("element")) -> (w172:u32[])
              n103 = disable-structure shown="Enabled" {
                disable-tunnel: w173 -> [w199 _]
                disable-tunnel: w172 -> [w198 w200]
                disable-tunnel: [w197 w200] -> w171
                frame Disabled {
                  n104 = Build Array (concatenate)(w199, w198) -> (w197:u32[])
                }
                frame Enabled {
                }
              }
            }
            frame "Circle" {
              # "Enabled This 1-23-2023"
              n105 = flat-sequence {
                tunnel: [w293] -> w280
                tunnel: w275 -> [w294]
                tunnel: w262 -> [w295]
                tunnel: w264 -> [w296]
                tunnel: w263 -> [w292]
                tunnel: [w291] -> w258
                tunnel: [w310] -> w286
                tunnel: [w309] -> w281
                tunnel: w280 -> [w309]
                tunnel: [w308] -> w259
                tunnel: w258 -> [w308]
                tunnel: w286 -> [w320]
                tunnel: [w320] -> w285
                tunnel: w281 -> [w318]
                tunnel: [w317] -> w279
                tunnel: w266 -> [w316]
                tunnel: w265 -> [w315]
                tunnel: [w319] -> w260
                tunnel: w259 -> [w319]
                tunnel: [w314] -> w255
                tunnel: [w313] -> w252
                tunnel: w285 -> [w327]
                tunnel: [w326] -> w283
                tunnel: [w325] -> w271
                tunnel: w279 -> [w324]
                tunnel: [w324] -> w278
                tunnel: [w323] -> w261
                tunnel: w260 -> [w323]
                tunnel: [w322] -> w256
                tunnel: w255 -> [w322]
                tunnel: [w321] -> w253
                tunnel: w252 -> [w321]
                tunnel: [w337] -> w284
                tunnel: w283 -> [w337]
                tunnel: w278 -> [w336]
                tunnel: [w335] -> w276
                tunnel: w274 -> [w329]
                tunnel: w273 -> [w334]
                tunnel: w272 -> [w331]
                tunnel: w261 -> [w330]
                tunnel: [w333] -> w257
                tunnel: w256 -> [w333]
                tunnel: [w332] -> w254
                tunnel: w253 -> [w332]
                tunnel: w284 -> [w342]
                tunnel: [w341] -> w270
                tunnel: [w340] -> w277
                tunnel: w276 -> [w340]
                tunnel: w257 -> [w339]
                tunnel: w254 -> [w338]
                tunnel: [w339] -> w251
                tunnel: [w338] -> w250
                tunnel: [w348] -> w282
                tunnel: w277 -> [w349]
                tunnel: w251 -> [w350]
                tunnel: w250 -> [w347]
                frame #0 {
                  n106 = case shown="True" w296 {
                    tunnel: w295 -> [w297 w305]
                    tunnel: w294 -> [w302 w307]
                    tunnel: [w301 w306] -> w293
                    tunnel: w292 -> [w300 _]
                    tunnel: [w299 w304] -> w291
                    frame False {
                      n107 = call "XY Go.vi"("return immediately"=FALSE, "Speed"=w300, "XY In"=w297, "Gantry In"=w302) -> ("XY Out"=w299:dbl[], "Gantry Out"=w301:refnum<k24>)  [unwired: 5 in, 1 out]
                    }
                    frame True {
                      n108 = call "ClearXYZTheta Go.vi"("Speed"=300.0, "XYZTheta In"=w305, "Gantry In"=w307) -> ("XYZTheta Out"=w304:dbl[], "Gantry Out"=w306:refnum<k24>)  [unwired: 6 in, 1 out]
                    }
                  }
                }
                frame #1 {
                  n109 = Tick Count (ms)() -> (millisecond timer value=w310:u32)
                }
                frame #2 {
                  n110 = call "Z Go.vi"("Increment"=TRUE, "Return Immediately"=FALSE, "Speed In"=w315, "Position In"=w316, "Gantry In"=w318) -> ("Speed Out"=w313:dbl, "Position Out"=w314:dbl, "Gantry Out"=w317:refnum<k24>)  [unwired: 3 in, 1 out]
                }
                frame #3 {
                  n111 = Tick Count (ms)() -> (millisecond timer value=w326:u32)
                  n112 = Subtract(x=w326, y=w327) -> (x-y=w325:u32)
                }
                frame #4 {
                  n113 = call "Circular.vi"("Direction"=w331, "return immediately"=FALSE, "Speed"=w334, "XY End"=w330, "XY Center"=w329, "Gantry In"=w336) -> ("Gantry Out"=w335:refnum<k24>)  [unwired: 4 in, 1 out]
                }
                frame #5 {
                  n114 = Tick Count (ms)() -> (millisecond timer value=w343:u32)
                  n115 = Subtract(x=w343, y=w342) -> (x-y=w341:u32)
                }
                frame #6 {
                  n116 = Negate(x=w350) -> (-x=w346:dbl)
                  n117 = call "Z Go.vi"("Increment"=TRUE, "Return Immediately"=FALSE, "Speed In"=w347, "Position In"=w346, "Gantry In"=w349) -> ("Gantry Out"=w348:refnum<k24>)  [unwired: 3 in, 3 out]
                }
              }
              n118 = Delete From Array(array=w249, length=1, index=0) -> (array with subset deleted=w248:T3)  [unwired: 1 out]
              n119 = Build Array(w271, w270) -> (w268:u32[])
              n120 = disable-structure shown="Enabled" {
                disable-tunnel: w269 -> [w289 _]
                disable-tunnel: w268 -> [w288 w290]
                disable-tunnel: [w287 w290] -> w267
                frame Enabled {
                  n121 = Build Array (concatenate)(w289, w288) -> (w287:u32[])
                }
                frame Disabled {
                }
              }
            }
            frame "Arc" {
              # "ENABLED THIS - 1/18/2023"
              n122 = flat-sequence {
                tunnel: w400 -> [w410]
                tunnel: w399 -> [w409]
                tunnel: w398 -> [w408]
                tunnel: [w407] -> w391
                tunnel: w377 -> [w406]
                tunnel: [w405] -> w361
                tunnel: w360 -> [w405]
                tunnel: w391 -> [w422]
                tunnel: [w422] -> w390
                tunnel: [w421] -> w388
                tunnel: [w420] -> w362
                tunnel: w361 -> [w420]
                tunnel: w390 -> [w432]
                tunnel: [w429] -> w393
                tunnel: w395 -> [w431]
                tunnel: w394 -> [w430]
                tunnel: [w428] -> w389
                tunnel: w388 -> [w428]
                tunnel: [w427] -> w385
                tunnel: [w426] -> w383
                tunnel: [w423] -> w363
                tunnel: w362 -> [w423]
                tunnel: w393 -> [w439]
                tunnel: [w439] -> w392
                tunnel: w389 -> [w438]
                tunnel: [w437] -> w386
                tunnel: w385 -> [w437]
                tunnel: [w436] -> w384
                tunnel: w383 -> [w436]
                tunnel: [w435] -> w382
                tunnel: [w434] -> w368
                tunnel: [w433] -> w364
                tunnel: w363 -> [w433]
                tunnel: w392 -> [w460]
                tunnel: w397 -> [w459]
                tunnel: w396 -> [w458]
                tunnel: w386 -> [w454]
                tunnel: w384 -> [w453]
                tunnel: w375 -> [w457]
                tunnel: w376 -> [w456]
                tunnel: [w455] -> w373
                tunnel: [w454] -> w371
                tunnel: [w453] -> w369
                tunnel: w368 -> [w452]
                tunnel: [w452] -> w367
                tunnel: w366 -> [w451]
                tunnel: [w450] -> w365
                tunnel: w364 -> [w449]
                tunnel: w359 -> [w448]
                tunnel: w358 -> [w446]
                tunnel: w357 -> [w447]
                tunnel: w356 -> [w445]
                tunnel: w355 -> [w444]
                tunnel: w354 -> [w443]
                tunnel: w353 -> [w442]
                tunnel: w352 -> [w441]
                tunnel: w351 -> [w440]
                tunnel: [w562] -> w381
                tunnel: [w561] -> w374
                tunnel: w373 -> [w561]
                tunnel: [w560] -> w372
                tunnel: w371 -> [w560]
                tunnel: [w559] -> w370
                tunnel: w369 -> [w559]
                tunnel: w367 -> [w557]
                tunnel: [w569] -> w387
                tunnel: w374 -> [w567]
                tunnel: w372 -> [w566]
                tunnel: w370 -> [w565]
                frame #0 {
                  n123 = case shown="True" w406 {
                    tunnel: [w415 w419] -> w407
                    tunnel: w410 -> [w414 w418]
                    tunnel: w409 -> [w411 w417]
                    tunnel: w408 -> [w413 _]
                    frame False {
                      n124 = call "XY Go.vi"("return immediately"=FALSE, "Speed"=w413, "XY In"=w411, "Gantry In"=w414) -> ("Gantry Out"=w415:refnum<k24>)  [unwired: 5 in, 2 out]
                    }
                    frame True {
                      n125 = call "ClearXYZTheta Go.vi"("Speed"=300.0, "XYZTheta In"=w417, "Gantry In"=w418) -> ("Gantry Out"=w419:refnum<k24>)  [unwired: 6 in, 2 out]
                    }
                  }
                }
                frame #1 {
                  n126 = Tick Count (ms)() -> (millisecond timer value=w421:u32)
                }
                frame #2 {
                  n127 = call "Z Go.vi"("Increment"=TRUE, "Return Immediately"=FALSE, "Speed In"=w430, "Position In"=w431, "Gantry In"=w432) -> ("Speed Out"=w426:dbl, "Position Out"=w427:dbl, "Gantry Out"=w429:refnum<k24>)  [unwired: 3 in, 1 out]
                }
                frame #3 {
                  n128 = Tick Count (ms)() -> (millisecond timer value=w434:u32)
                  n129 = Subtract(x=w434, y=w438) -> (x-y=w435:u32)
                }
                frame #4 {
                  n130 = case shown="True" w447 {
                    tunnel: w460 -> [w472 w556]
                    tunnel: w459 -> [w470 w555]
                    tunnel: w458 -> [w475 w554]
                    tunnel: w457 -> [w474 w553]
                    tunnel: w456 -> [w473 w552]
                    tunnel: [w471 w551] -> w455
                    tunnel: w451 -> [w477 w547]
                    tunnel: [w476 w546] -> w450
                    tunnel: w449 -> [w469 _]
                    tunnel: w448 -> [w468 _]
                    tunnel: w446 -> [w467 _]
                    tunnel: w445 -> [w466 _]
                    tunnel: w444 -> [w465 _]
                    tunnel: w443 -> [w464 _]
                    tunnel: w442 -> [w463 _]
                    tunnel: w441 -> [w462 _]
                    tunnel: w440 -> [w461 _]
                    frame True {
                      # "direction"
                      # "center"
                      # "end"
                      n131 = case shown="True" w467 {
                        tunnel: w477 -> [w479 w545]
                        tunnel: [w478 w542] -> w476
                        tunnel: w475 -> [w493 w541]
                        tunnel: w474 -> [w488 w534]
                        tunnel: w473 -> [w489 w533]
                        tunnel: w472 -> [w491 w540]
                        tunnel: [w490 w538] -> w471
                        tunnel: w470 -> [w492 w537]
                        tunnel: w469 -> [w487 _]
                        tunnel: w468 -> [w486 _]
                        tunnel: w466 -> [w485 w532]
                        tunnel: w465 -> [w484 w531]
                        tunnel: w464 -> [w483 _]
                        tunnel: w463 -> [w482 _]
                        tunnel: w462 -> [w481 _]
                        tunnel: w461 -> [w480 _]
                        frame True {
                          n132 = case shown="True" w487 {
                            tunnel: w493 -> [w505 w530]
                            tunnel: w492 -> [w506 w515]
                            tunnel: w491 -> [w510 w523]
                            tunnel: [w507 w519] -> w490
                            tunnel: w489 -> [w504 w528]
                            tunnel: w488 -> [w503 w529]
                            tunnel: w486 -> [_ _]
                            tunnel: w485 -> [w501 w526]
                            tunnel: w484 -> [w500 w527]
                            tunnel: w483 -> [w499 w525]
                            tunnel: w482 -> [w498 w524]
                            tunnel: w481 -> [_ w518]
                            tunnel: w480 -> [_ w517]
                            tunnel: w479 -> [w495 w514]
                            tunnel: [w494 w513] -> w478
                            frame False {
                              w502 = FALSE
                              n133 = call "Circular.vi"("Direction"=w505, "return immediately"=w502, "Speed"=w506, "XY End"=w504, "XY Center"=w503, "Gantry In"=w510) -> ("Gantry Out"=w509:refnum<k24>)  [unwired: 4 in, 1 out]
                              n134 = call "Circular.vi"("Direction"=w505, "return immediately"=w502, "Speed"=w506, "XY End"=w500, "XY Center"=w501, "Gantry In"=w509) -> ("Gantry Out"=w508:refnum<k24>)  [unwired: 4 in, 1 out]
                              n135 = call "Circular.vi"("Direction"=w505, "return immediately"=w502, "Speed"=w506, "XY End"=w499, "XY Center"=w498, "Gantry In"=w508) -> ("Gantry Out"=w507:refnum<k24>)  [unwired: 4 in, 1 out]
                              n136 = Delete From Array(array=w495, length=3, index=0) -> (array with subset deleted=w494:T3)  [unwired: 1 out]
                            }
                            frame True {
                              w516 = FALSE
                              n137 = Delete From Array(array=w514, length=4, index=0) -> (array with subset deleted=w513:T3)  [unwired: 1 out]
                              n138 = call "Circular.vi"("Direction"=w530, "return immediately"=w516, "Speed"=w515, "XY End"=w528, "XY Center"=w529, "Gantry In"=w523) -> ("Gantry Out"=w522:refnum<k24>)  [unwired: 4 in, 1 out]
                              n139 = call "Circular.vi"("Direction"=w530, "return immediately"=w516, "Speed"=w515, "XY End"=w527, "XY Center"=w526, "Gantry In"=w522) -> ("Gantry Out"=w521:refnum<k24>)  [unwired: 4 in, 1 out]
                              n140 = call "Circular.vi"("Direction"=w530, "return immediately"=w516, "Speed"=w515, "XY End"=w525, "XY Center"=w524, "Gantry In"=w521) -> ("Gantry Out"=w520:refnum<k24>)  [unwired: 4 in, 1 out]
                              n141 = call "Circular.vi"("Direction"=w530, "return immediately"=w516, "Speed"=w515, "XY End"=w518, "XY Center"=w517, "Gantry In"=w520) -> ("Gantry Out"=w519:refnum<k24>)  [unwired: 4 in, 1 out]
                            }
                          }
                        }
                        frame False {
                          n142 = call "Circular.vi"("Direction"=w541, "return immediately"=FALSE, "Speed"=w537, "XY End"=w533, "XY Center"=w534, "Gantry In"=w540) -> ("Gantry Out"=w539:refnum<k24>)  [unwired: 4 in, 1 out]
                          n143 = call "Circular.vi"("Direction"=w541, "return immediately"=FALSE, "Speed"=w537, "XY End"=w531, "XY Center"=w532, "Gantry In"=w539) -> ("Gantry Out"=w538:refnum<k24>)  [unwired: 4 in, 1 out]
                          n144 = Delete From Array(array=w545, length=2, index=0) -> (array with subset deleted=w542:T3)  [unwired: 1 out]
                        }
                      }
                    }
                    frame False {
                      # "end"
                      # "center"
                      # "direction"
                      n145 = call "Circular.vi"("Direction"=w554, "return immediately"=FALSE, "Speed"=w555, "XY End"=w552, "XY Center"=w553, "Gantry In"=w556) -> ("Gantry Out"=w551:refnum<k24>)  [unwired: 4 in, 1 out]
                      n146 = Delete From Array(array=w547, length=1, index=0) -> (array with subset deleted=w546:T3)  [unwired: 1 out]
                    }
                  }
                }
                frame #5 {
                  n147 = Tick Count (ms)() -> (millisecond timer value=w558:u32)
                  n148 = Subtract(x=w558, y=w557) -> (x-y=w562:u32)
                }
                frame #6 {
                  n149 = Negate(x=w566) -> (-x=w568:dbl)
                  n150 = call "Z Go.vi"("Increment"=TRUE, "Return Immediately"=FALSE, "Speed In"=w565, "Position In"=w568, "Gantry In"=w567) -> ("Gantry Out"=w569:refnum<k24>)  [unwired: 3 in, 3 out]
                }
              }
              n151 = Build Array "Build Array"(w382, w381) -> (w380:u32[])
              n152 = disable-structure shown="Enabled" {
                disable-tunnel: w380 -> [w403 w404]
                disable-tunnel: w379 -> [w402 _]
                disable-tunnel: [w401 w404] -> w378
                frame Enabled {
                  n153 = Build Array (concatenate) "Build Array"(w403, w402) -> (w401:u32[])
                }
                frame Disabled {
                }
              }
            }
            frame "Line" {
              n154 = flat-sequence {
                tunnel: w629 -> [w638]
                tunnel: w628 -> [w634]
                tunnel: w627 -> [w637]
                tunnel: w626 -> [w636]
                tunnel: [w635] -> w625
                tunnel: w625 -> [w648]
                tunnel: [w648] -> w624
                tunnel: [w649] -> w620
                tunnel: w624 -> [w658]
                tunnel: w623 -> [w657]
                tunnel: w622 -> [w656]
                tunnel: [w655] -> w621
                tunnel: w620 -> [w655]
                tunnel: [w654] -> w618
                tunnel: [w653] -> w609
                tunnel: [w652] -> w605
                tunnel: w621 -> [w664]
                tunnel: [w663] -> w602
                tunnel: [w662] -> w619
                tunnel: w618 -> [w662]
                tunnel: [w661] -> w615
                tunnel: [w660] -> w610
                tunnel: w609 -> [w660]
                tunnel: [w659] -> w606
                tunnel: w605 -> [w659]
                tunnel: w619 -> [w698]
                tunnel: w617 -> [w697]
                tunnel: [w696] -> w616
                tunnel: w615 -> [w696]
                tunnel: [w695] -> w613
                tunnel: [w694] -> w611
                tunnel: w610 -> [w694]
                tunnel: [w693] -> w607
                tunnel: w606 -> [w693]
                tunnel: w598 -> [w692]
                tunnel: w597 -> [w691]
                tunnel: w596 -> [w690]
                tunnel: w595 -> [w687]
                tunnel: w594 -> [w689]
                tunnel: [w688] -> w593
                tunnel: w592 -> [w686]
                tunnel: w591 -> [w685]
                tunnel: w590 -> [w684]
                tunnel: w589 -> [_]
                tunnel: w588 -> [w683]
                tunnel: w587 -> [w682]
                tunnel: w586 -> [w681]
                tunnel: w585 -> [w680]
                tunnel: w584 -> [w679]
                tunnel: w583 -> [w678]
                tunnel: w582 -> [w677]
                tunnel: w581 -> [w676]
                tunnel: w580 -> [w675]
                tunnel: w579 -> [w674]
                tunnel: w578 -> [w673]
                tunnel: w577 -> [w672]
                tunnel: w576 -> [w671]
                tunnel: w575 -> [w670]
                tunnel: w574 -> [w669]
                tunnel: w573 -> [w668]
                tunnel: w572 -> [w667]
                tunnel: w571 -> [w666]
                tunnel: w570 -> [w665]
                tunnel: w616 -> [w1235]
                tunnel: [w1234] -> w604
                tunnel: [w1233] -> w614
                tunnel: w613 -> [w1233]
                tunnel: [w1232] -> w612
                tunnel: w611 -> [w1232]
                tunnel: [w1231] -> w608
                tunnel: w607 -> [w1231]
                tunnel: w614 -> [w1243]
                tunnel: w612 -> [w1242]
                tunnel: w608 -> [w1240]
                tunnel: [w1239] -> w603
                frame #0 {
                  n155 = case shown="True" w636 {
                    tunnel: w638 -> [w643 w647]
                    tunnel: w637 -> [w642 _]
                    tunnel: [w641 w646] -> w635
                    tunnel: w634 -> [w640 w645]
                    frame False {
                      n156 = call "XY Go.vi"("return immediately"=FALSE, "Speed"=w642, "XY In"=w640, "Gantry In"=w643) -> ("Gantry Out"=w641:refnum<k24>)  [unwired: 5 in, 2 out]
                    }
                    frame True {
                      n157 = call "ClearXYZTheta Go.vi"("Speed"=300.0, "XYZTheta In"=w645, "Gantry In"=w647) -> ("Gantry Out"=w646:refnum<k24>)  [unwired: 6 in, 2 out]
                    }
                  }
                }
                frame #1 {
                  n158 = Tick Count (ms)() -> (millisecond timer value=w649:u32)
                }
                frame #2 {
                  # "ok"
                  n159 = call "Z Go.vi"("Increment"=TRUE, "Return Immediately"=FALSE, "Speed In"=w656, "Position In"=w657, "Gantry In"=w658) -> ("Speed Out"=w652:dbl, "Position Out"=w653:dbl, "Gantry Out"=w654:refnum<k24>)  [unwired: 3 in, 1 out]
                }
                frame #3 {
                  n160 = Tick Count (ms)() -> (millisecond timer value=w661:u32)
                  n161 = Subtract(x=w661, y=w664) -> (x-y=w663:u32)
                }
                frame #4 {
                  n162 = case shown="True" w691 {
                    tunnel: w698 -> [w705 w737]
                    tunnel: w697 -> [w707 w736]
                    tunnel: [w704 w735] -> w695
                    tunnel: w692 -> [w706 w734]
                    tunnel: w690 -> [_ w733]
                    tunnel: w687 -> [_ w732]
                    tunnel: w689 -> [w702 w731]
                    tunnel: [w701 w730] -> w688
                    tunnel: w686 -> [_ w729]
                    tunnel: w685 -> [_ w728]
                    tunnel: w684 -> [_ w727]
                    tunnel: w683 -> [_ w726]
                    tunnel: w682 -> [_ w725]
                    tunnel: w681 -> [_ w724]
                    tunnel: w680 -> [_ w723]
                    tunnel: w679 -> [_ w722]
                    tunnel: w678 -> [_ w721]
                    tunnel: w677 -> [_ w720]
                    tunnel: w676 -> [_ w719]
                    tunnel: w675 -> [_ w718]
                    tunnel: w674 -> [_ w717]
                    tunnel: w673 -> [_ w716]
                    tunnel: w672 -> [_ w715]
                    tunnel: w671 -> [_ w714]
                    tunnel: w670 -> [_ w713]
                    tunnel: w669 -> [_ w712]
                    tunnel: w668 -> [_ w711]
                    tunnel: w667 -> [_ w710]
                    tunnel: w666 -> [_ w709]
                    tunnel: w665 -> [_ w708]
                    frame False {
                      n163 = call "XY Go.vi"("return immediately"=FALSE, "Speed"=w707, "XY In"=w706, "Gantry In"=w705) -> ("Gantry Out"=w704:refnum<k24>)  [unwired: 5 in, 2 out]
                      n164 = Delete From Array(array=w702, length=1, index=0) -> (array with subset deleted=w701:T3)  [unwired: 1 out]
                    }
                    frame True {
                      n165 = case shown="True" w733 {
                        tunnel: w737 -> [w749 w775]
                        tunnel: w736 -> [w747 w777]
                        tunnel: [w744 w774] -> w735
                        tunnel: w734 -> [w748 w776]
                        tunnel: w732 -> [_ _]
                        tunnel: w731 -> [w743 w773]
                        tunnel: [w742 w772] -> w730
                        tunnel: w729 -> [w738 w771]
                        tunnel: w728 -> [_ w770]
                        tunnel: w727 -> [_ w769]
                        tunnel: w726 -> [_ w768]
                        tunnel: w725 -> [_ w767]
                        tunnel: w724 -> [_ w766]
                        tunnel: w723 -> [_ w765]
                        tunnel: w722 -> [_ w764]
                        tunnel: w721 -> [_ w763]
                        tunnel: w720 -> [_ w762]
                        tunnel: w719 -> [_ w761]
                        tunnel: w718 -> [_ w760]
                        tunnel: w717 -> [_ w759]
                        tunnel: w716 -> [_ w758]
                        tunnel: w715 -> [_ w757]
                        tunnel: w714 -> [_ w756]
                        tunnel: w713 -> [_ w755]
                        tunnel: w712 -> [_ w754]
                        tunnel: w711 -> [_ w753]
                        tunnel: w710 -> [_ w752]
                        tunnel: w709 -> [_ w751]
                        tunnel: w708 -> [_ w750]
                        frame False {
                          n166 = Delete From Array(array=w743, length=2, index=0) -> (array with subset deleted=w742:T3)  [unwired: 1 out]
                          n167 = call "XY Go.vi"("return immediately"=FALSE, "Speed"=w747, "XY In"=w748, "Gantry In"=w749) -> ("Gantry Out"=w745:refnum<k24>)  [unwired: 5 in, 2 out]
                          n168 = call "XY Go.vi"("return immediately"=FALSE, "Speed"=w747, "XY In"=w738, "Gantry In"=w745) -> ("Gantry Out"=w744:refnum<k24>)  [unwired: 5 in, 2 out]
                        }
                        frame True {
                          # "#8"
                          # "#7"
                          # "#6"
                          # "#5"
                          # "#4"
                          # "#3"
                          # "#1"
                          # "#2"
                          n169 = case shown="True" w769 {
                            tunnel: w777 -> [w779 w812]
                            tunnel: w776 -> [w790 w813]
                            tunnel: w775 -> [w789 w815]
                            tunnel: [w781 w814] -> w774
                            tunnel: w773 -> [w788 w817]
                            tunnel: [w787 w816] -> w772
                            tunnel: w771 -> [w780 w811]
                            tunnel: w770 -> [w778 w810]
                            tunnel: w768 -> [_ w809]
                            tunnel: w767 -> [_ w808]
                            tunnel: w766 -> [_ w807]
                            tunnel: w765 -> [_ w806]
                            tunnel: w764 -> [_ w805]
                            tunnel: w763 -> [_ w804]
                            tunnel: w762 -> [_ w803]
                            tunnel: w761 -> [_ w802]
                            tunnel: w760 -> [_ w801]
                            tunnel: w759 -> [_ w800]
                            tunnel: w758 -> [_ w799]
                            tunnel: w757 -> [_ w798]
                            tunnel: w756 -> [_ w797]
                            tunnel: w755 -> [_ w796]
                            tunnel: w754 -> [_ w795]
                            tunnel: w753 -> [_ w794]
                            tunnel: w752 -> [_ w793]
                            tunnel: w751 -> [_ w792]
                            tunnel: w750 -> [_ w791]
                            frame False {
                              n170 = call "XY Go.vi"("return immediately"=FALSE, "Speed"=w779, "XY In"=w790, "Gantry In"=w789) -> ("Gantry Out"=w783:refnum<k24>)  [unwired: 5 in, 2 out]
                              n171 = call "XY Go.vi"("Speed"=w779, "XY In"=w780, "Gantry In"=w783) -> ("Gantry Out"=w782:refnum<k24>)  [unwired: 6 in, 2 out]
                              n172 = Delete From Array(array=w788, length=3, index=0) -> (array with subset deleted=w787:T3)  [unwired: 1 out]
                              n173 = call "XY Go.vi"("Speed"=w779, "XY In"=w778, "Gantry In"=w782) -> ("Gantry Out"=w781:refnum<k24>)  [unwired: 6 in, 2 out]
                            }
                            frame True {
                              n174 = case shown="True" w792 {
                                tunnel: [w821 w858] -> w816
                                tunnel: w817 -> [w822 w857]
                                tunnel: w815 -> [w832 w856]
                                tunnel: [w828 w855] -> w814
                                tunnel: w813 -> [w827 w853]
                                tunnel: w812 -> [w826 w854]
                                tunnel: w811 -> [w825 w852]
                                tunnel: w810 -> [w824 w851]
                                tunnel: w809 -> [w823 w850]
                                tunnel: w808 -> [_ w849]
                                tunnel: w807 -> [_ w848]
                                tunnel: w806 -> [_ w847]
                                tunnel: w805 -> [_ w846]
                                tunnel: w804 -> [_ w845]
                                tunnel: w803 -> [_ w844]
                                tunnel: w802 -> [_ w843]
                                tunnel: w801 -> [_ w842]
                                tunnel: w800 -> [_ w841]
                                tunnel: w799 -> [_ w840]
                                tunnel: w798 -> [_ w839]
                                tunnel: w797 -> [_ w838]
                                tunnel: w796 -> [_ w837]
                                tunnel: w795 -> [_ w836]
                                tunnel: w794 -> [_ w835]
                                tunnel: w793 -> [_ w834]
                                tunnel: w791 -> [_ w833]
                                frame False {
                                w818 = FALSE
                                n175 = call "XY Go.vi"("return immediately"=w818, "Speed"=w826, "XY In"=w827, "Gantry In"=w832) -> ("Gantry Out"=w831:refnum<k24>)  [unwired: 5 in, 2 out]
                                n176 = Delete From Array(array=w822, length=4, index=0) -> (array with subset deleted=w821:T3)  [unwired: 1 out]
                                n177 = call "XY Go.vi"("return immediately"=w818, "Speed"=w826, "XY In"=w825, "Gantry In"=w831) -> ("Gantry Out"=w830:refnum<k24>)  [unwired: 5 in, 2 out]
                                n178 = call "XY Go.vi"("return immediately"=w818, "Speed"=w826, "XY In"=w824, "Gantry In"=w830) -> ("Gantry Out"=w829:refnum<k24>)  [unwired: 5 in, 2 out]
                                n179 = call "XY Go.vi"("return immediately"=w818, "Speed"=w826, "XY In"=w823, "Gantry In"=w829) -> ("Gantry Out"=w828:refnum<k24>)  [unwired: 5 in, 2 out]
                                }
                                frame True {
                                n180 = case shown="True" w833 {
                                tunnel: [w874 w897] -> w858
                                tunnel: w857 -> [w875 w898]
                                tunnel: w856 -> [w871 w900]
                                tunnel: [w866 w899] -> w855
                                tunnel: w854 -> [w861 w896]
                                tunnel: w853 -> [w865 w895]
                                tunnel: w852 -> [w864 w894]
                                tunnel: w851 -> [w863 w892]
                                tunnel: w850 -> [w862 w893]
                                tunnel: w849 -> [w860 w891]
                                tunnel: w848 -> [_ w890]
                                tunnel: w847 -> [_ w889]
                                tunnel: w846 -> [_ w888]
                                tunnel: w845 -> [_ w887]
                                tunnel: w844 -> [_ w886]
                                tunnel: w843 -> [_ w885]
                                tunnel: w842 -> [_ w884]
                                tunnel: w841 -> [_ w883]
                                tunnel: w840 -> [_ w882]
                                tunnel: w839 -> [_ w881]
                                tunnel: w838 -> [_ w880]
                                tunnel: w837 -> [_ w879]
                                tunnel: w836 -> [_ w878]
                                tunnel: w835 -> [_ w877]
                                tunnel: w834 -> [_ w876]
                                frame False {
                                w859 = FALSE
                                n181 = call "XY Go.vi"("return immediately"=w859, "Speed"=w861, "XY In"=w865, "Gantry In"=w871) -> ("Gantry Out"=w870:refnum<k24>)  [unwired: 5 in, 2 out]
                                n182 = Delete From Array(array=w875, length=5, index=0) -> (array with subset deleted=w874:T3)  [unwired: 1 out]
                                n183 = call "XY Go.vi"("return immediately"=w859, "Speed"=w861, "XY In"=w864, "Gantry In"=w870) -> ("Gantry Out"=w869:refnum<k24>)  [unwired: 5 in, 2 out]
                                n184 = call "XY Go.vi"("return immediately"=w859, "Speed"=w861, "XY In"=w863, "Gantry In"=w869) -> ("Gantry Out"=w868:refnum<k24>)  [unwired: 5 in, 2 out]
                                n185 = call "XY Go.vi"("return immediately"=w859, "Speed"=w861, "XY In"=w862, "Gantry In"=w868) -> ("Gantry Out"=w867:refnum<k24>)  [unwired: 5 in, 2 out]
                                n186 = call "XY Go.vi"("return immediately"=w859, "Speed"=w861, "XY In"=w860, "Gantry In"=w867) -> ("Gantry Out"=w866:refnum<k24>)  [unwired: 5 in, 2 out]
                                }
                                frame True {
                                n187 = case shown="True" w876 {
                                tunnel: w900 -> [w919 w941]
                                tunnel: [w913 w940] -> w899
                                tunnel: w898 -> [w910 w943]
                                tunnel: [w909 w939] -> w897
                                tunnel: w896 -> [w908 w938]
                                tunnel: w895 -> [w907 w942]
                                tunnel: w894 -> [w906 w937]
                                tunnel: w893 -> [w905 w920]
                                tunnel: w892 -> [w904 w921]
                                tunnel: w891 -> [w903 w936]
                                tunnel: w890 -> [w902 w935]
                                tunnel: w889 -> [_ w934]
                                tunnel: w888 -> [_ w933]
                                tunnel: w887 -> [_ w932]
                                tunnel: w886 -> [_ w931]
                                tunnel: w885 -> [_ w930]
                                tunnel: w884 -> [_ w929]
                                tunnel: w883 -> [_ w928]
                                tunnel: w882 -> [_ w927]
                                tunnel: w881 -> [_ w926]
                                tunnel: w880 -> [_ w925]
                                tunnel: w879 -> [_ w924]
                                tunnel: w878 -> [_ w923]
                                tunnel: w877 -> [_ w922]
                                frame False {
                                w901 = FALSE
                                n188 = call "XY Go.vi"("return immediately"=w901, "Speed"=w908, "XY In"=w907, "Gantry In"=w919) -> ("Gantry Out"=w918:refnum<k24>)  [unwired: 5 in, 2 out]
                                n189 = call "XY Go.vi"("return immediately"=w901, "Speed"=w908, "XY In"=w906, "Gantry In"=w918) -> ("Gantry Out"=w917:refnum<k24>)  [unwired: 5 in, 2 out]
                                n190 = call "XY Go.vi"("return immediately"=w901, "Speed"=w908, "XY In"=w905, "Gantry In"=w917) -> ("Gantry Out"=w916:refnum<k24>)  [unwired: 5 in, 2 out]
                                n191 = Delete From Array(array=w910, length=6, index=0) -> (array with subset deleted=w909:T3)  [unwired: 1 out]
                                n192 = call "XY Go.vi"("return immediately"=w901, "Speed"=w908, "XY In"=w904, "Gantry In"=w916) -> ("Gantry Out"=w915:refnum<k24>)  [unwired: 5 in, 2 out]
                                n193 = call "XY Go.vi"("return immediately"=w901, "Speed"=w908, "XY In"=w903, "Gantry In"=w915) -> ("Gantry Out"=w914:refnum<k24>)  [unwired: 5 in, 2 out]
                                n194 = call "XY Go.vi"("return immediately"=w901, "Speed"=w908, "XY In"=w902, "Gantry In"=w914) -> ("Gantry Out"=w913:refnum<k24>)  [unwired: 5 in, 2 out]
                                }
                                frame True {
                                # "#5"
                                # "#4"
                                n195 = case shown="True" w927 {
                                tunnel: w943 -> [w963 w986]
                                tunnel: w942 -> [w960 w981]
                                tunnel: w941 -> [w959 w984]
                                tunnel: [w952 w983] -> w940
                                tunnel: [w951 w985] -> w939
                                tunnel: w938 -> [w950 w982]
                                tunnel: w937 -> [w949 w980]
                                tunnel: w920 -> [w945 w979]
                                tunnel: w921 -> [w944 w978]
                                tunnel: w936 -> [w948 w977]
                                tunnel: w935 -> [w947 w976]
                                tunnel: w934 -> [w946 w975]
                                tunnel: w933 -> [_ w974]
                                tunnel: w932 -> [_ w973]
                                tunnel: w931 -> [_ w972]
                                tunnel: w930 -> [_ w971]
                                tunnel: w929 -> [_ w970]
                                tunnel: w928 -> [_ w969]
                                tunnel: w926 -> [_ w968]
                                tunnel: w925 -> [_ w967]
                                tunnel: w924 -> [_ w966]
                                tunnel: w923 -> [_ w965]
                                tunnel: w922 -> [_ w964]
                                frame False {
                                n196 = call "XY Go.vi"("Speed"=w950, "XY In"=w960, "Gantry In"=w959) -> ("Gantry Out"=w958:refnum<k24>)  [unwired: 6 in, 2 out]
                                n197 = call "XY Go.vi"("Speed"=w950, "XY In"=w949, "Gantry In"=w958) -> ("Gantry Out"=w957:refnum<k24>)  [unwired: 6 in, 2 out]
                                n198 = call "XY Go.vi"("Speed"=w950, "XY In"=w944, "Gantry In"=w957) -> ("Gantry Out"=w956:refnum<k24>)  [unwired: 6 in, 2 out]
                                n199 = Delete From Array(array=w963, length=7, index=0) -> (array with subset deleted=w951:T3)  [unwired: 1 out]
                                n200 = call "XY Go.vi"("Speed"=w950, "XY In"=w945, "Gantry In"=w956) -> ("Gantry Out"=w955:refnum<k24>)  [unwired: 6 in, 2 out]
                                n201 = call "XY Go.vi"("Speed"=w950, "XY In"=w948, "Gantry In"=w955) -> ("Gantry Out"=w954:refnum<k24>)  [unwired: 6 in, 2 out]
                                n202 = call "XY Go.vi"("Speed"=w950, "XY In"=w947, "Gantry In"=w954) -> ("Gantry Out"=w953:refnum<k24>)  [unwired: 6 in, 2 out]
                                n203 = call "XY Go.vi"("Speed"=w950, "XY In"=w946, "Gantry In"=w953) -> ("Gantry Out"=w952:refnum<k24>)  [unwired: 6 in, 2 out]
                                }
                                frame True {
                                n204 = case shown="True" w968 {
                                tunnel: w986 -> [w1008 w1030]
                                tunnel: [w1007 w1027] -> w985
                                tunnel: w984 -> [w1004 w1029]
                                tunnel: [w996 w1028] -> w983
                                tunnel: w982 -> [w995 w1026]
                                tunnel: w981 -> [w994 w1025]
                                tunnel: w980 -> [w993 w1024]
                                tunnel: w979 -> [w987 w1023]
                                tunnel: w978 -> [w988 w1022]
                                tunnel: w977 -> [w992 w1021]
                                tunnel: w976 -> [w991 w1020]
                                tunnel: w975 -> [w990 w1019]
                                tunnel: w974 -> [w989 w1018]
                                tunnel: w973 -> [_ w1017]
                                tunnel: w972 -> [_ w1016]
                                tunnel: w971 -> [_ w1015]
                                tunnel: w970 -> [_ w1014]
                                tunnel: w969 -> [_ w1013]
                                tunnel: w967 -> [_ w1012]
                                tunnel: w966 -> [_ w1011]
                                tunnel: w965 -> [_ w1010]
                                tunnel: w964 -> [_ w1009]
                                frame False {
                                n205 = call "XY Go.vi"("Speed"=w995, "XY In"=w994, "Gantry In"=w1004) -> ("Gantry Out"=w1003:refnum<k24>)  [unwired: 6 in, 2 out]
                                n206 = call "XY Go.vi"("Speed"=w995, "XY In"=w993, "Gantry In"=w1003) -> ("Gantry Out"=w1002:refnum<k24>)  [unwired: 6 in, 2 out]
                                n207 = call "XY Go.vi"("Speed"=w995, "XY In"=w988, "Gantry In"=w1002) -> ("Gantry Out"=w1001:refnum<k24>)  [unwired: 6 in, 2 out]
                                n208 = Delete From Array(array=w1008, length=8, index=0) -> (array with subset deleted=w1007:T3)  [unwired: 1 out]
                                n209 = call "XY Go.vi"("Speed"=w995, "XY In"=w987, "Gantry In"=w1001) -> ("Gantry Out"=w1000:refnum<k24>)  [unwired: 6 in, 2 out]
                                n210 = call "XY Go.vi"("Speed"=w995, "XY In"=w992, "Gantry In"=w1000) -> ("Gantry Out"=w999:refnum<k24>)  [unwired: 6 in, 2 out]
                                n211 = call "XY Go.vi"("Speed"=w995, "XY In"=w991, "Gantry In"=w999) -> ("Gantry Out"=w998:refnum<k24>)  [unwired: 6 in, 2 out]
                                n212 = call "XY Go.vi"("Speed"=w995, "XY In"=w990, "Gantry In"=w998) -> ("Gantry Out"=w997:refnum<k24>)  [unwired: 6 in, 2 out]
                                n213 = call "XY Go.vi"("Speed"=w995, "XY In"=w989, "Gantry In"=w997) -> ("Gantry Out"=w996:refnum<k24>)  [unwired: 6 in, 2 out]
                                }
                                frame True {
                                # "#11"
                                # "#10"
                                # "#9"
                                n214 = case shown="True" w1012 {
                                tunnel: w1030 -> [w1054 w1075]
                                tunnel: w1029 -> [w1051 w1073]
                                tunnel: [w1042 w1072] -> w1028
                                tunnel: [w1041 w1074] -> w1027
                                tunnel: w1026 -> [w1040 w1071]
                                tunnel: w1025 -> [w1039 w1070]
                                tunnel: w1024 -> [w1038 w1069]
                                tunnel: w1023 -> [w1031 w1068]
                                tunnel: w1022 -> [w1032 w1067]
                                tunnel: w1021 -> [w1037 w1066]
                                tunnel: w1020 -> [w1036 w1065]
                                tunnel: w1019 -> [w1035 w1064]
                                tunnel: w1018 -> [w1034 w1063]
                                tunnel: w1017 -> [w1033 w1062]
                                tunnel: w1016 -> [_ w1061]
                                tunnel: w1015 -> [_ w1060]
                                tunnel: w1014 -> [_ w1059]
                                tunnel: w1013 -> [_ w1058]
                                tunnel: w1011 -> [_ w1057]
                                tunnel: w1010 -> [_ w1056]
                                tunnel: w1009 -> [_ w1055]
                                frame False {
                                n215 = call "XY Go.vi"("Speed"=w1040, "XY In"=w1039, "Gantry In"=w1051) -> ("Gantry Out"=w1050:refnum<k24>)  [unwired: 6 in, 2 out]
                                n216 = call "XY Go.vi"("Speed"=w1040, "XY In"=w1038, "Gantry In"=w1050) -> ("Gantry Out"=w1049:refnum<k24>)  [unwired: 6 in, 2 out]
                                n217 = call "XY Go.vi"("Speed"=w1040, "XY In"=w1032, "Gantry In"=w1049) -> ("Gantry Out"=w1048:refnum<k24>)  [unwired: 6 in, 2 out]
                                n218 = call "XY Go.vi"("Speed"=w1040, "XY In"=w1031, "Gantry In"=w1048) -> ("Gantry Out"=w1047:refnum<k24>)  [unwired: 6 in, 2 out]
                                n219 = Delete From Array(array=w1054, length=9, index=0) -> (array with subset deleted=w1041:T3)  [unwired: 1 out]
                                n220 = call "XY Go.vi"("Speed"=w1040, "XY In"=w1037, "Gantry In"=w1047) -> ("Gantry Out"=w1046:refnum<k24>)  [unwired: 6 in, 2 out]
                                n221 = call "XY Go.vi"("Speed"=w1040, "XY In"=w1036, "Gantry In"=w1046) -> ("Gantry Out"=w1045:refnum<k24>)  [unwired: 6 in, 2 out]
                                n222 = call "XY Go.vi"("Speed"=w1040, "XY In"=w1035, "Gantry In"=w1045) -> ("Gantry Out"=w1044:refnum<k24>)  [unwired: 6 in, 2 out]
                                n223 = call "XY Go.vi"("Speed"=w1040, "XY In"=w1034, "Gantry In"=w1044) -> ("Gantry Out"=w1043:refnum<k24>)  [unwired: 6 in, 2 out]
                                n224 = call "XY Go.vi"("Speed"=w1040, "XY In"=w1033, "Gantry In"=w1043) -> ("Gantry Out"=w1042:refnum<k24>)  [unwired: 6 in, 2 out]
                                }
                                frame True {
                                n225 = case shown="True" w1057 {
                                tunnel: w1075 -> [w1101 w1121]
                                tunnel: [w1100 w1120] -> w1074
                                tunnel: w1073 -> [w1097 w1116]
                                tunnel: [w1087 w1115] -> w1072
                                tunnel: w1071 -> [w1086 w1118]
                                tunnel: w1070 -> [w1085 w1119]
                                tunnel: w1069 -> [w1084 w1117]
                                tunnel: w1068 -> [w1077 w1114]
                                tunnel: w1067 -> [w1076 w1113]
                                tunnel: w1066 -> [w1083 w1112]
                                tunnel: w1065 -> [w1082 w1111]
                                tunnel: w1064 -> [w1081 w1110]
                                tunnel: w1063 -> [w1080 w1109]
                                tunnel: w1062 -> [w1079 w1108]
                                tunnel: w1061 -> [w1078 w1107]
                                tunnel: w1060 -> [_ w1106]
                                tunnel: w1059 -> [_ w1105]
                                tunnel: w1058 -> [_ w1104]
                                tunnel: w1056 -> [_ w1103]
                                tunnel: w1055 -> [_ w1102]
                                frame False {
                                n226 = call "XY Go.vi"("Speed"=w1086, "XY In"=w1085, "Gantry In"=w1097) -> ("Gantry Out"=w1096:refnum<k24>)  [unwired: 6 in, 2 out]
                                n227 = call "XY Go.vi"("Speed"=w1086, "XY In"=w1084, "Gantry In"=w1096) -> ("Gantry Out"=w1095:refnum<k24>)  [unwired: 6 in, 2 out]
                                n228 = call "XY Go.vi"("Speed"=w1086, "XY In"=w1076, "Gantry In"=w1095) -> ("Gantry Out"=w1094:refnum<k24>)  [unwired: 6 in, 2 out]
                                n229 = call "XY Go.vi"("Speed"=w1086, "XY In"=w1077, "Gantry In"=w1094) -> ("Gantry Out"=w1093:refnum<k24>)  [unwired: 6 in, 2 out]
                                n230 = Delete From Array(array=w1101, length=10, index=0) -> (array with subset deleted=w1100:T3)  [unwired: 1 out]
                                n231 = call "XY Go.vi"("Speed"=w1086, "XY In"=w1083, "Gantry In"=w1093) -> ("Gantry Out"=w1092:refnum<k24>)  [unwired: 6 in, 2 out]
                                n232 = call "XY Go.vi"("Speed"=w1086, "XY In"=w1082, "Gantry In"=w1092) -> ("Gantry Out"=w1091:refnum<k24>)  [unwired: 6 in, 2 out]
                                n233 = call "XY Go.vi"("Speed"=w1086, "XY In"=w1081, "Gantry In"=w1091) -> ("Gantry Out"=w1090:refnum<k24>)  [unwired: 6 in, 2 out]
                                n234 = call "XY Go.vi"("Speed"=w1086, "XY In"=w1080, "Gantry In"=w1090) -> ("Gantry Out"=w1089:refnum<k24>)  [unwired: 6 in, 2 out]
                                n235 = call "XY Go.vi"("Speed"=w1086, "XY In"=w1079, "Gantry In"=w1089) -> ("Gantry Out"=w1088:refnum<k24>)  [unwired: 6 in, 2 out]
                                n236 = call "XY Go.vi"("Speed"=w1086, "XY In"=w1078, "Gantry In"=w1088) -> ("Gantry Out"=w1087:refnum<k24>)  [unwired: 6 in, 2 out]
                                }
                                frame True {
                                n237 = case shown="True" w1103 {
                                tunnel: w1121 -> [w1147 w1168]
                                tunnel: [w1146 w1167] -> w1120
                                tunnel: w1119 -> [w1145 w1166]
                                tunnel: w1118 -> [w1131 w1163]
                                tunnel: w1117 -> [w1144 w1162]
                                tunnel: w1116 -> [w1143 w1165]
                                tunnel: [w1132 w1164] -> w1115
                                tunnel: w1114 -> [w1123 w1150]
                                tunnel: w1113 -> [w1122 w1151]
                                tunnel: w1112 -> [w1130 w1161]
                                tunnel: w1111 -> [w1129 w1160]
                                tunnel: w1110 -> [w1128 w1159]
                                tunnel: w1109 -> [w1127 w1158]
                                tunnel: w1108 -> [w1126 w1157]
                                tunnel: w1107 -> [w1125 w1156]
                                tunnel: w1106 -> [w1124 w1155]
                                tunnel: w1105 -> [_ w1154]
                                tunnel: w1104 -> [_ w1153]
                                tunnel: w1102 -> [_ w1152]
                                frame False {
                                n238 = call "XY Go.vi"("Speed"=w1131, "XY In"=w1145, "Gantry In"=w1143) -> ("Gantry Out"=w1142:refnum<k24>)  [unwired: 6 in, 2 out]
                                n239 = call "XY Go.vi"("Speed"=w1131, "XY In"=w1144, "Gantry In"=w1142) -> ("Gantry Out"=w1141:refnum<k24>)  [unwired: 6 in, 2 out]
                                n240 = call "XY Go.vi"("Speed"=w1131, "XY In"=w1122, "Gantry In"=w1141) -> ("Gantry Out"=w1140:refnum<k24>)  [unwired: 6 in, 2 out]
                                n241 = call "XY Go.vi"("Speed"=w1131, "XY In"=w1123, "Gantry In"=w1140) -> ("Gantry Out"=w1139:refnum<k24>)  [unwired: 6 in, 2 out]
                                n242 = call "XY Go.vi"("Speed"=w1131, "XY In"=w1130, "Gantry In"=w1139) -> ("Gantry Out"=w1138:refnum<k24>)  [unwired: 6 in, 2 out]
                                n243 = Delete From Array(array=w1147, length=11, index=0) -> (array with subset deleted=w1146:T3)  [unwired: 1 out]
                                n244 = call "XY Go.vi"("Speed"=w1131, "XY In"=w1129, "Gantry In"=w1138) -> ("Gantry Out"=w1137:refnum<k24>)  [unwired: 6 in, 2 out]
                                n245 = call "XY Go.vi"("Speed"=w1131, "XY In"=w1128, "Gantry In"=w1137) -> ("Gantry Out"=w1136:refnum<k24>)  [unwired: 6 in, 2 out]
                                n246 = call "XY Go.vi"("Speed"=w1131, "XY In"=w1127, "Gantry In"=w1136) -> ("Gantry Out"=w1135:refnum<k24>)  [unwired: 6 in, 2 out]
                                n247 = call "XY Go.vi"("Speed"=w1131, "XY In"=w1126, "Gantry In"=w1135) -> ("Gantry Out"=w1134:refnum<k24>)  [unwired: 6 in, 2 out]
                                n248 = call "XY Go.vi"("Speed"=w1131, "XY In"=w1125, "Gantry In"=w1134) -> ("Gantry Out"=w1133:refnum<k24>)  [unwired: 6 in, 2 out]
                                n249 = call "XY Go.vi"("Speed"=w1131, "XY In"=w1124, "Gantry In"=w1133) -> ("Gantry Out"=w1132:refnum<k24>)  [unwired: 6 in, 2 out]
                                }
                                frame True {
                                n250 = case shown="True" w1152 {
                                tunnel: w1168 -> [w1198 w1228]
                                tunnel: [w1197 w1227] -> w1167
                                tunnel: w1166 -> [w1194 w1226]
                                tunnel: w1165 -> [w1193 w1225]
                                tunnel: [w1181 w1212] -> w1164
                                tunnel: w1163 -> [w1180 w1202]
                                tunnel: w1162 -> [w1179 w1211]
                                tunnel: w1161 -> [w1178 w1210]
                                tunnel: w1160 -> [w1177 w1209]
                                tunnel: w1159 -> [w1176 w1208]
                                tunnel: w1158 -> [w1175 w1207]
                                tunnel: w1157 -> [w1174 w1206]
                                tunnel: w1156 -> [w1173 w1205]
                                tunnel: w1155 -> [w1172 w1204]
                                tunnel: w1154 -> [w1171 w1203]
                                tunnel: w1153 -> [_ w1201]
                                tunnel: w1150 -> [w1170 w1200]
                                tunnel: w1151 -> [w1169 w1199]
                                frame False {
                                n251 = call "XY Go.vi"("Speed"=w1180, "XY In"=w1194, "Gantry In"=w1193) -> ("Gantry Out"=w1192:refnum<k24>)  [unwired: 6 in, 2 out]
                                n252 = call "XY Go.vi"("Speed"=w1180, "XY In"=w1179, "Gantry In"=w1192) -> ("Gantry Out"=w1191:refnum<k24>)  [unwired: 6 in, 2 out]
                                n253 = call "XY Go.vi"("Speed"=w1180, "XY In"=w1169, "Gantry In"=w1191) -> ("Gantry Out"=w1190:refnum<k24>)  [unwired: 6 in, 2 out]
                                n254 = call "XY Go.vi"("Speed"=w1180, "XY In"=w1170, "Gantry In"=w1190) -> ("Gantry Out"=w1189:refnum<k24>)  [unwired: 6 in, 2 out]
                                n255 = Delete From Array(array=w1198, length=12, index=0) -> (array with subset deleted=w1197:T3)  [unwired: 1 out]
                                n256 = call "XY Go.vi"("Speed"=w1180, "XY In"=w1178, "Gantry In"=w1189) -> ("Gantry Out"=w1188:refnum<k24>)  [unwired: 6 in, 2 out]
                                n257 = call "XY Go.vi"("Speed"=w1180, "XY In"=w1177, "Gantry In"=w1188) -> ("Gantry Out"=w1187:refnum<k24>)  [unwired: 6 in, 2 out]
                                n258 = call "XY Go.vi"("Speed"=w1180, "XY In"=w1176, "Gantry In"=w1187) -> ("Gantry Out"=w1186:refnum<k24>)  [unwired: 6 in, 2 out]
                                n259 = call "XY Go.vi"("Speed"=w1180, "XY In"=w1175, "Gantry In"=w1186) -> ("Gantry Out"=w1185:refnum<k24>)  [unwired: 6 in, 2 out]
                                n260 = call "XY Go.vi"("Speed"=w1180, "XY In"=w1174, "Gantry In"=w1185) -> ("Gantry Out"=w1184:refnum<k24>)  [unwired: 6 in, 2 out]
                                n261 = call "XY Go.vi"("Speed"=w1180, "XY In"=w1173, "Gantry In"=w1184) -> ("Gantry Out"=w1183:refnum<k24>)  [unwired: 6 in, 2 out]
                                n262 = call "XY Go.vi"("Speed"=w1180, "XY In"=w1172, "Gantry In"=w1183) -> ("Gantry Out"=w1182:refnum<k24>)  [unwired: 6 in, 2 out]
                                n263 = call "XY Go.vi"("Speed"=w1180, "XY In"=w1171, "Gantry In"=w1182) -> ("Gantry Out"=w1181:refnum<k24>)  [unwired: 6 in, 2 out]
                                }
                                frame True {
                                n264 = call "XY Go.vi"("Speed"=w1202, "XY In"=w1226, "Gantry In"=w1225) -> ("Gantry Out"=w1224:refnum<k24>)  [unwired: 6 in, 2 out]
                                n265 = call "XY Go.vi"("Speed"=w1202, "XY In"=w1211, "Gantry In"=w1224) -> ("Gantry Out"=w1223:refnum<k24>)  [unwired: 6 in, 2 out]
                                n266 = call "XY Go.vi"("Speed"=w1202, "XY In"=w1199, "Gantry In"=w1223) -> ("Gantry Out"=w1222:refnum<k24>)  [unwired: 6 in, 2 out]
                                n267 = call "XY Go.vi"("Speed"=w1202, "XY In"=w1200, "Gantry In"=w1222) -> ("Gantry Out"=w1221:refnum<k24>)  [unwired: 6 in, 2 out]
                                n268 = call "XY Go.vi"("Speed"=w1202, "XY In"=w1210, "Gantry In"=w1221) -> ("Gantry Out"=w1220:refnum<k24>)  [unwired: 6 in, 2 out]
                                n269 = call "XY Go.vi"("Speed"=w1202, "XY In"=w1209, "Gantry In"=w1220) -> ("Gantry Out"=w1219:refnum<k24>)  [unwired: 6 in, 2 out]
                                n270 = Delete From Array(array=w1228, length=13, index=0) -> (array with subset deleted=w1227:T3)  [unwired: 1 out]
                                n271 = call "XY Go.vi"("Speed"=w1202, "XY In"=w1208, "Gantry In"=w1219) -> ("Gantry Out"=w1218:refnum<k24>)  [unwired: 6 in, 2 out]
                                n272 = call "XY Go.vi"("Speed"=w1202, "XY In"=w1207, "Gantry In"=w1218) -> ("Gantry Out"=w1217:refnum<k24>)  [unwired: 6 in, 2 out]
                                n273 = call "XY Go.vi"("Speed"=w1202, "XY In"=w1206, "Gantry In"=w1217) -> ("Gantry Out"=w1216:refnum<k24>)  [unwired: 6 in, 2 out]
                                n274 = call "XY Go.vi"("Speed"=w1202, "XY In"=w1205, "Gantry In"=w1216) -> ("Gantry Out"=w1215:refnum<k24>)  [unwired: 6 in, 2 out]
                                n275 = call "XY Go.vi"("Speed"=w1202, "XY In"=w1204, "Gantry In"=w1215) -> ("Gantry Out"=w1214:refnum<k24>)  [unwired: 6 in, 2 out]
                                n276 = call "XY Go.vi"("Speed"=w1202, "XY In"=w1203, "Gantry In"=w1214) -> ("Gantry Out"=w1213:refnum<k24>)  [unwired: 6 in, 2 out]
                                n277 = call "XY Go.vi"("Speed"=w1202, "XY In"=w1201, "Gantry In"=w1213) -> ("Gantry Out"=w1212:refnum<k24>)  [unwired: 6 in, 2 out]
                                }
                                }
                                }
                                }
                                }
                                }
                                }
                                }
                                }
                                }
                                }
                                }
                                }
                                }
                                }
                                }
                                }
                              }
                            }
                          }
                        }
                      }
                    }
                  }
                }
                frame #5 {
                  # "measures time\nit takes to move\nfrom P(i) to P(i+1)"
                  n278 = Tick Count (ms)() -> (millisecond timer value=w1236:u32)
                  n279 = Subtract(x=w1236, y=w1235) -> (x-y=w1234:u32)
                }
                frame #6 {
                  n280 = Negate(x=w1242) -> (-x=w1241:dbl)
                  n281 = call "Z Go.vi"("Increment"=TRUE, "Return Immediately"=FALSE, "Speed In"=w1240, "Position In"=w1241, "Gantry In"=w1243) -> ("Gantry Out"=w1239:refnum<k24>)  [unwired: 3 in, 3 out]
                }
              }
              n282 = Build Array(w602, w604) -> (w600:u32[])
              n283 = disable-structure shown="Enabled" {
                disable-tunnel: w601 -> [w632 _]
                disable-tunnel: w600 -> [w631 w633]
                disable-tunnel: [w630 w633] -> w599
                frame Disabled {
                  n284 = Build Array (concatenate)(w632, w631) -> (w630:u32[])
                }
                frame Enabled {
                }
              }
            }
          }
          n285 = Array Size(array=w115) -> (size(s)=w114:i32)
          n286 = Equal To 0?(x=w114) -> (x = 0?=w112:bool)
        }
        "Timing Data" <- w18
        n287 = in-place-cluster #1("Gantry"=w19) -> (w9:T2)
      }
    }
    frame Error {
      (unwired) T3 [] ("Dispense Steps")
    }
  }
  "error out" <- w2
  "Sensor Dispense out" <- w5
  "Control Out" <- w3
